vi "main_002.vi"() -> ()   [LabVIEW 2017]
uses:
  ISEGNHQxxu/iseg NHQ VISA Control.ctl
  <vilib>/Analysis/1siggen.llb/Ramp Pattern by Samples.vi
  <vilib>/Utility/file.llb/Read From Spreadsheet File (DBL).vi
  <vilib>/Utility/file.llb/Write Delimited Spreadsheet (string).vi
  <vilib>/Utility/file.llb/Write Delimited Spreadsheet (DBL).vi
  <vilib>/Platform/browser.llb/Open URL in Default Browser (path).vi
  <vilib>/Analysis/NI_AALBase.lvlib
  Newport ESP301/Newport ESP301.lvlib
panel:
  in  "continous acq.":bool
  in  "snap":bool
  in  "dark":bool
  in  "savebin":bool
  in  "savepng":bool
  in  "count?":bool
  in  "dark?":bool=TRUE
  in  "threshold":i32=300
  in  "t_exp":dbl=0.10000637173652649 caption="Exposure time [s]"
  in  "dark_load":bool
  in  "frames":i32=300
  in  "avg[t] acc[f]":bool
  in  "Value in":dbl=2.0 caption="binning"
  in  "stop":bool
  out "Slide":dbl(slide)=0.9966666666666667 scale=0.0..1.0
  in  "open base path":bool
  in  "Path":path=path "Z:/Ediff/data/2018/08/180807"
  in  "Tab Control":T1(tab)=enum."delayscan"
  out "Waveform Chart":dbl(graph)=8402498.700000005
  in  "array size":i32=50
  out "noise-o-meter":dbl=7.252741087138157 format="%.1g"
  out "Actual Voltage":dbl[unit]=-90.03 format="%.2f"
  in  "volt_set":bool
  in  "Nominal Voltage":sgl=90.0 min=0 max=1000 step=1 format="%.2f"
  in  "delayscan_go":bool
  in  "waypoints":string[][](table)=[["-500", "50"], ["500", ""], ["", ""]]
  in  "delayscan_header":string="DelayScan01" caption="header"
  in  "iterations":i32=1
  out "XY Graph":cluster{"Array":dbl[], dbl[]}(graph)={"Array"=[-500.0, -450.0, -400.0, -350.0, -300.0, -250.0, -200.0, -150.0, -100.0, -50.0, 0.0, 50.0, 100.0, 150.0, 200.0, 250.0, 300.0, 350.0, 400.0, 450.0, 500.0], [74.7680418855, 74.77553669695, 0.0, 0.0, 0.0, 0.0, 0.0, 0.0, 0.0, 0.0, 0.0, 0.0, 0.0, 0.0, 0.0, 0.0, 0.0, 0.0, 0.0, 0.0, 0.0]}
  in  "delayscan_stop":bool
  in  "esp_abs_dest":dbl=74.87296924580001 caption="[mm]"
  out "t0 @":dbl=74.84299 format="%.6g"
  in  "esp_set_t0":bool
  in  "esp_abs_time":dbl=200.0 caption="[fs]"
  in  "esp_rel_delta":dbl=0.015 caption="delta [mm]" min=0.0
  in  "esp_abs_go":bool
  in  "esp_rel-":bool
  in  "esp_rel+":bool
  out "delay_pos":dbl=74.77555 caption="[mm]" format="%.6g"
  out "esp_pos_fs":dbl=-449.91125160329966 caption="[fs]" format="%.6g"
  out "Slide 2":dbl(slide)=0.999 scale=0.0..1.0
  in  "meas_stop_volt":bool
  in  "meas_start_volt":bool
  in  "head":string="PowerVoltScan1"
  in  "volt_start":dbl format="%0.2f"
  in  "volt_end":dbl=1.0 format="%0.2f"
  in  "volt_samples":i32=128
  in  "move2com":bool
  in  "meas_start_XY":bool
  in  "showcom":bool
  in  "VISA ISEG":refnum<visa-resource-name>="COM3"
  in  "Channel (A)":enum16{"A", "B"}(ring)=enum."B"
  out "error out":errorcluster
  in  "volt_timeout":u32=6000
  in  "volt_threshold":sgl=2.0 max=4000 format="%.2f"
  in  "esp_axis":i32=1 caption="ESP Axis" min=1 max=3
  in  "esp_visa":refnum<visa-resource-name>="COM2" caption="ESP VISA"
  out "esp301":errorcluster
  in  "Serial Link (RS232)":enum16{"RS232", "USB"}(ring)
  out "captured":dbl[][](graph)
  out "live":dbl[][](graph)
  in  "close":bool
  # "camera"
  # "voltage supply"
  # "Move absolute"
  # "Move relative"
  # "Axis1"
  # "Axis2"
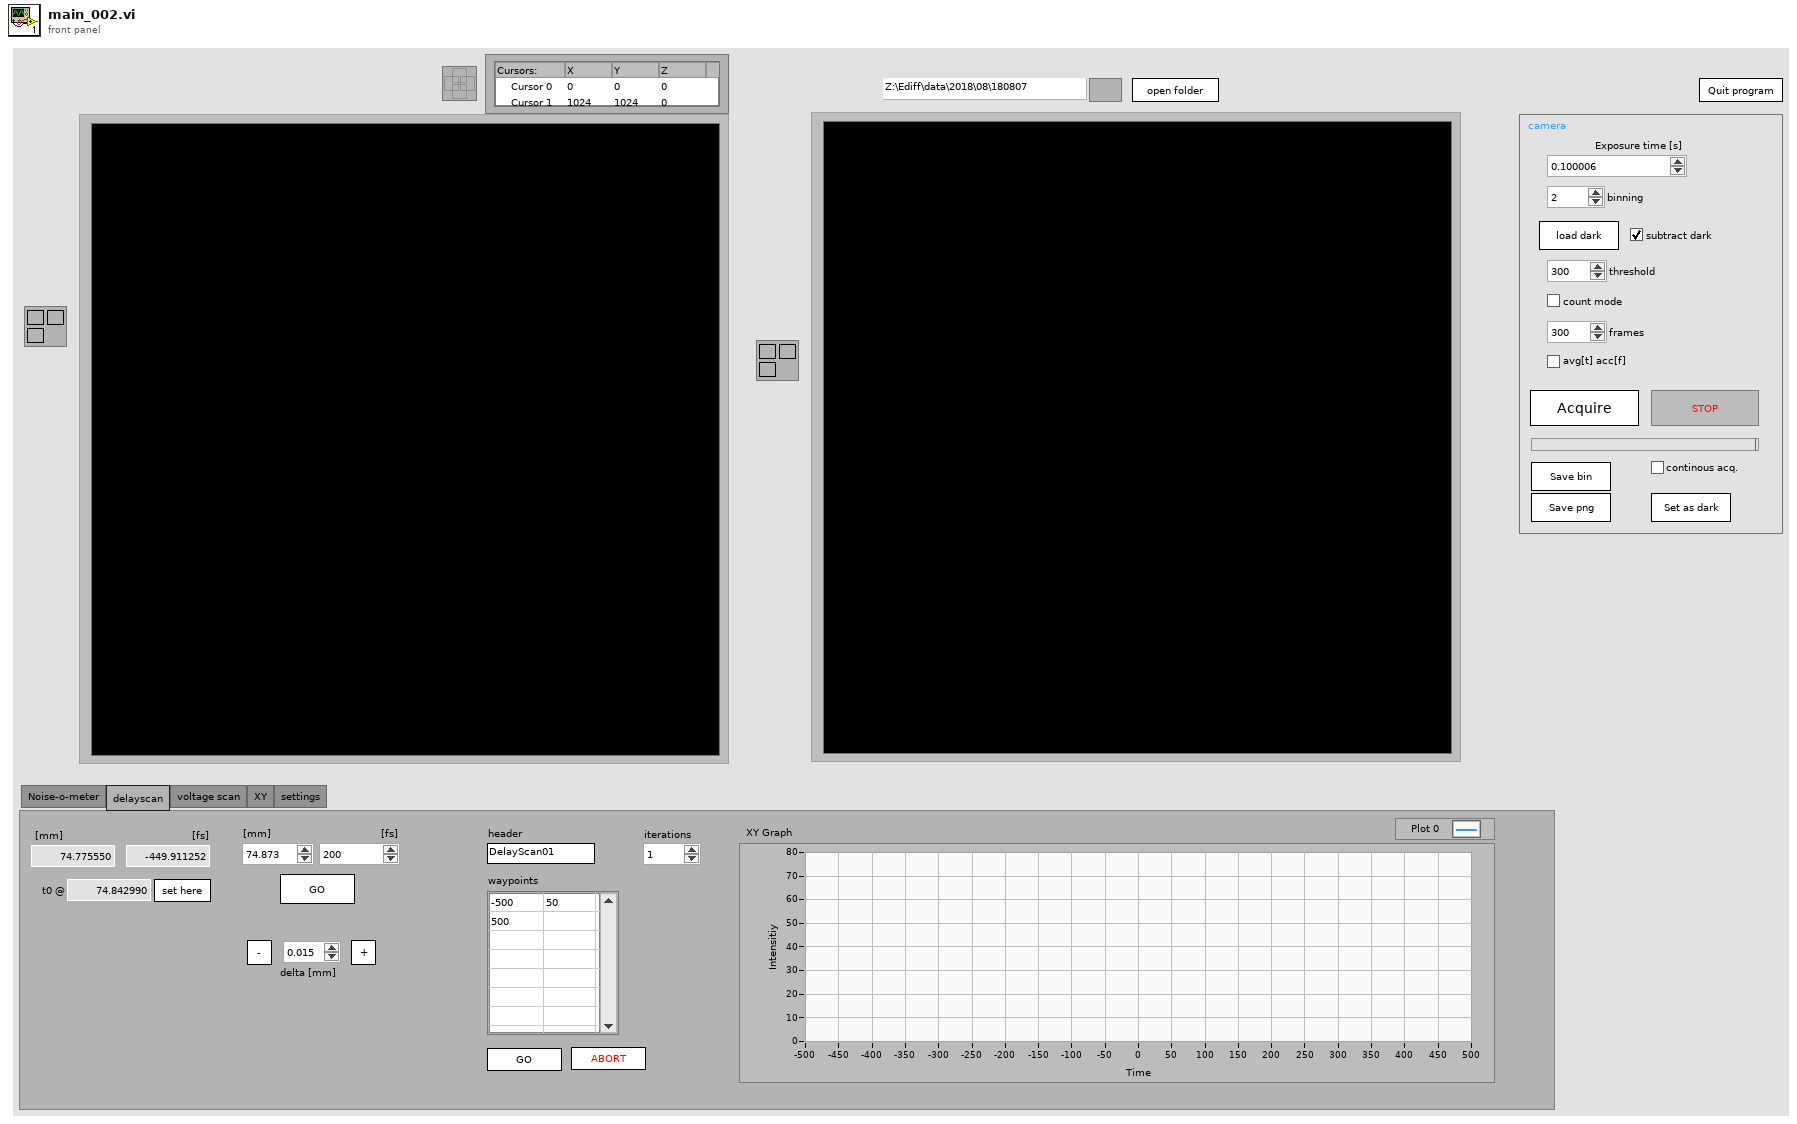
[diagram p1: front panel]
types:
  T1 = enum32{"Noise-o-meter", "delayscan", "voltage scan", "XY", "settings"}
  T2 = typedef "Image Type" = u32
  T3 = typedef "IMAQ Image.ctl" = refnum<image>
  T4 = cluster{"height":u32, "width":u32, "datatype":u32}
  T5 = cluster{"Axis1 moving":bool, "Axis2 moving":bool, "Axis3 moving":bool, "Axis4 moving":bool, "Motor Power of at least one axis":bool, "Reserved":bool, "Reserved":bool, "Reserved":bool, "Axis5 moving 2":bool, "Axis6 moving 2":bool, "Reserved":bool, "Reserved":bool, "Motor Power of at least one axis":bool, "Reserved":bool, "Reserved":bool, "Reserved":bool}
  T6 = typedef "iseg NHQ VISA Control.ctl" = cluster{"VISA Resource Name":refnum<visa-resource-name>, "FP Notation":bool, "Maximum Voltage":u32, "Maximum Current":u32}
  T7 = typedef "LVCursorListTypeDef.ctl" = cluster{"Name":string, "Color":u32, "Style":u8, "Point Style":u8, "Name Visible":bool, "Allow Drag":bool, "Cursor Mode":u32, "Plot":i32, "Index":i32, "Position":cluster{"X":dbl, "Y":dbl}, "X Scale":u32, "Y Scale":u32, "Watch Plots":i32[], "Watch All Plots":bool, "Plot Area":i32, "Label Offset":cluster{"X":dbl, "Y":dbl}}[]
  T8 = cluster{"Name":string, "Color":u32, "Style":u8, "Point Style":u8, "Name Visible":bool, "Allow Drag":bool, "Cursor Mode":u32, "Plot":i32, "Index":i32, "Position":cluster{"X":dbl, "Y":dbl}, "X Scale":u32, "Y Scale":u32, "Watch Plots":i32[], "Watch All Plots":bool, "Plot Area":i32, "Label Offset":cluster{"X":dbl, "Y":dbl}}
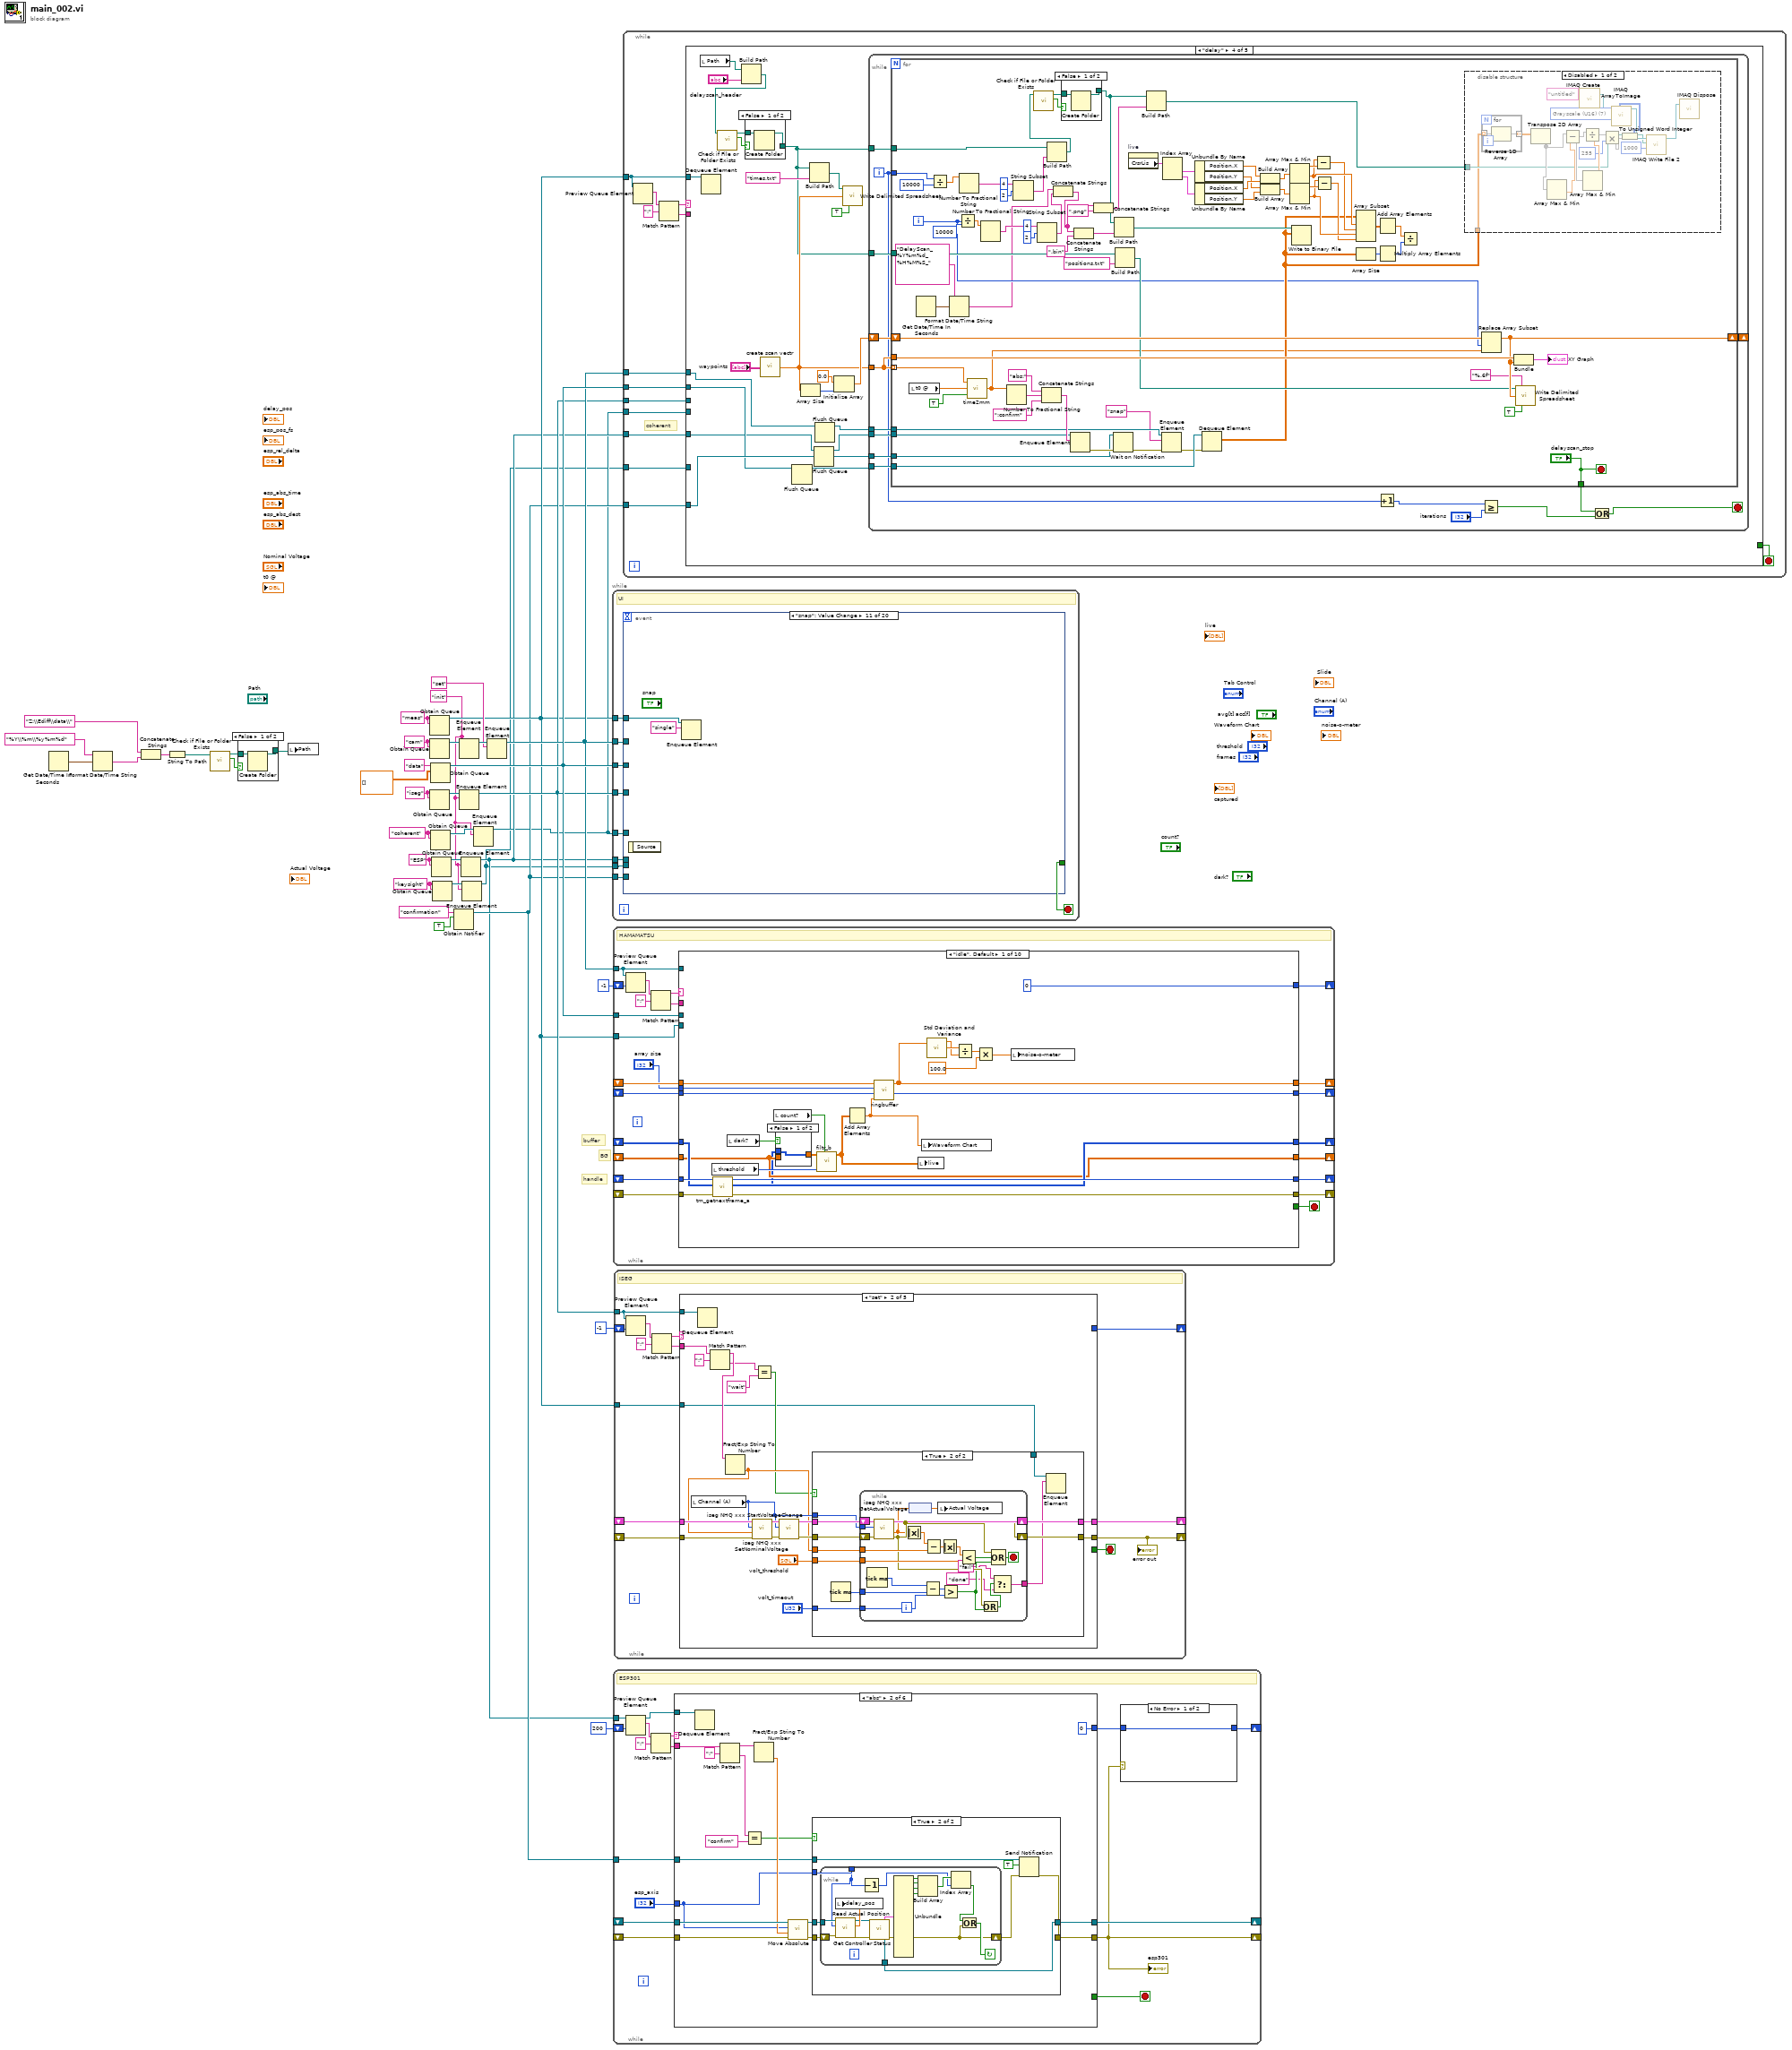
[diagram p0: block diagram]
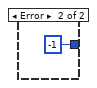
[diagram p3: hidden frame]
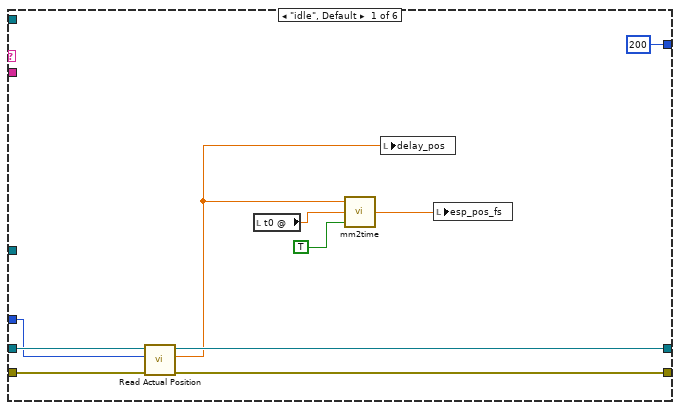
[diagram p4: hidden frame]
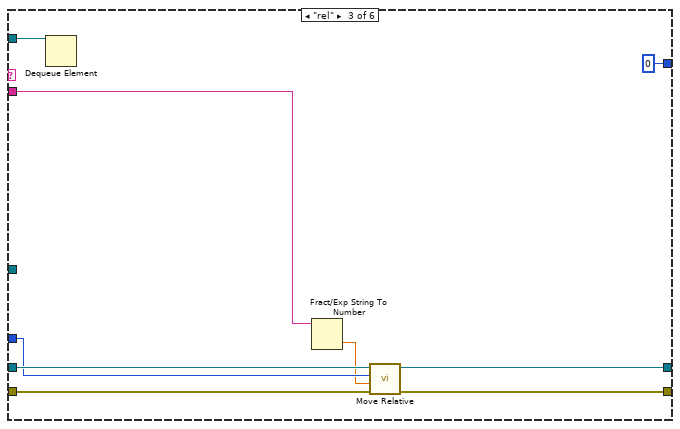
[diagram p6: hidden frame]
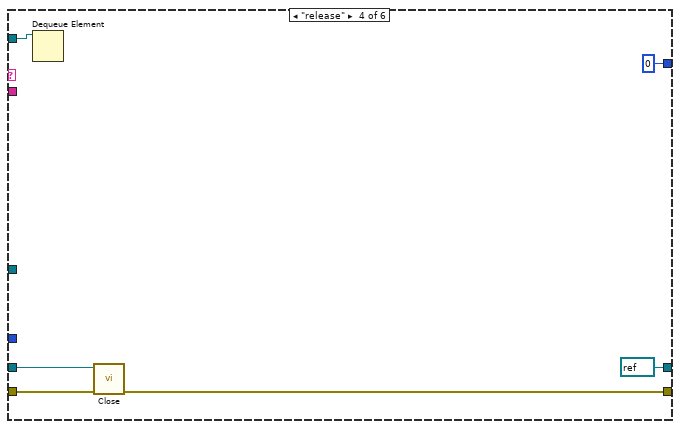
[diagram p7: hidden frame]
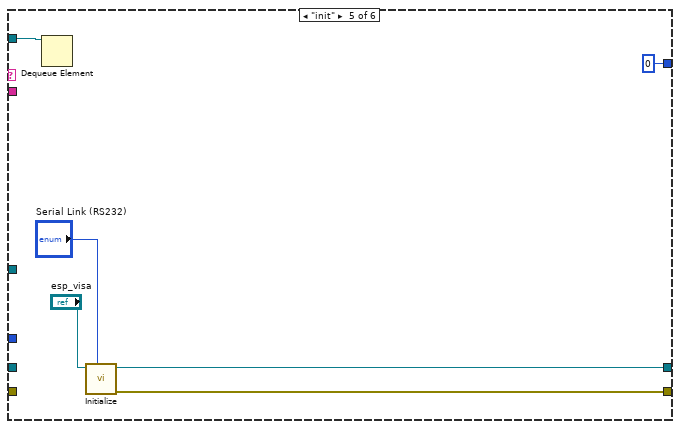
[diagram p8: hidden frame]
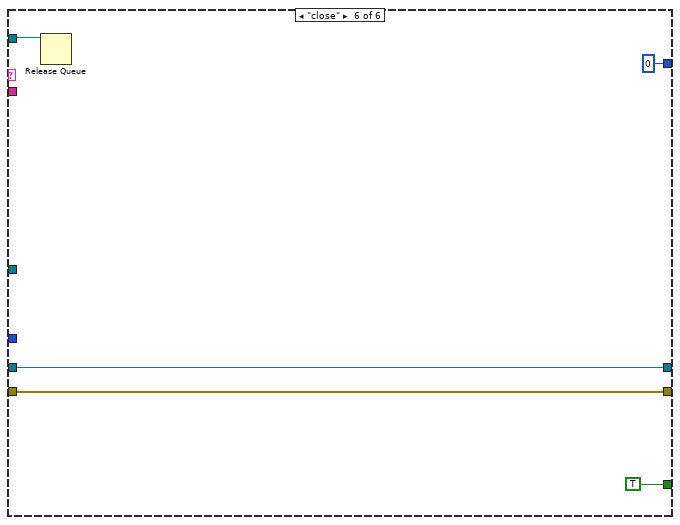
[diagram p9: hidden frame]
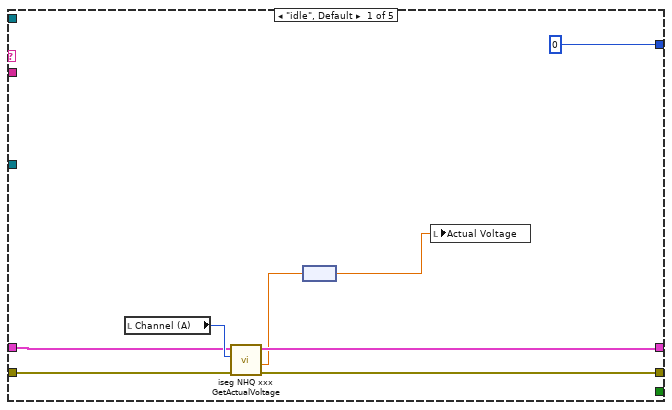
[diagram p10: hidden frame]
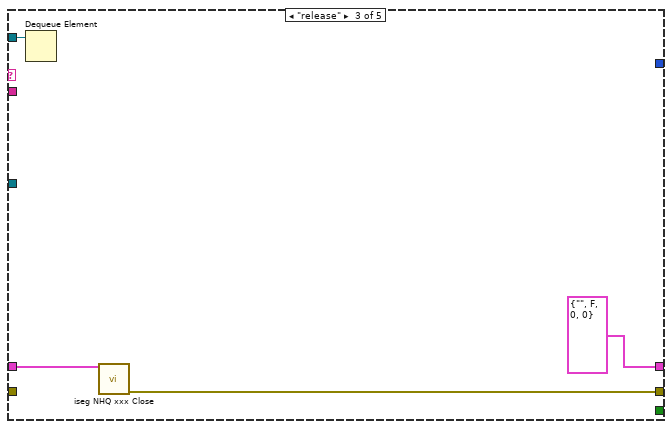
[diagram p12: hidden frame]
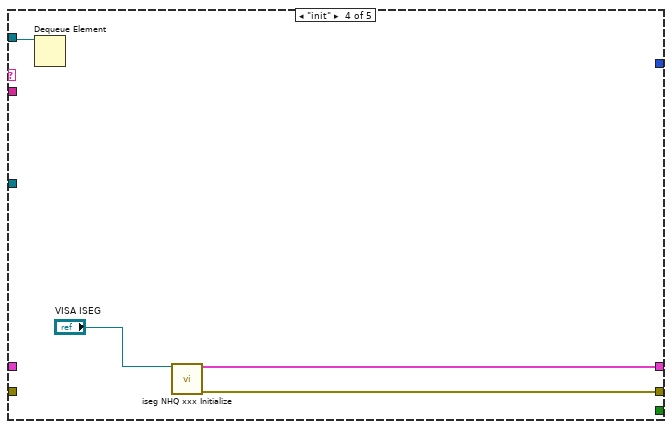
[diagram p13: hidden frame]
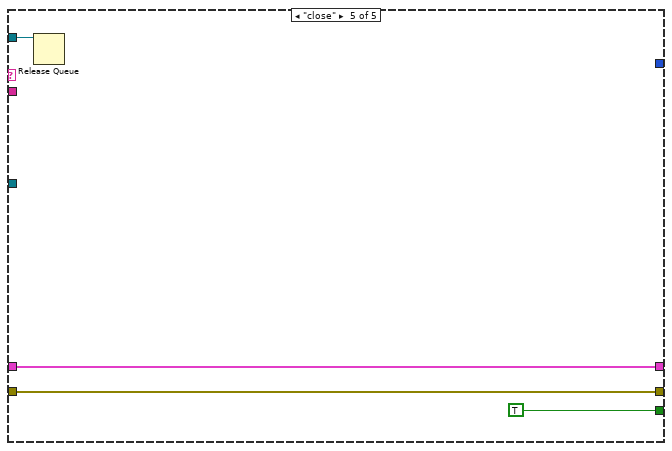
[diagram p14: hidden frame]
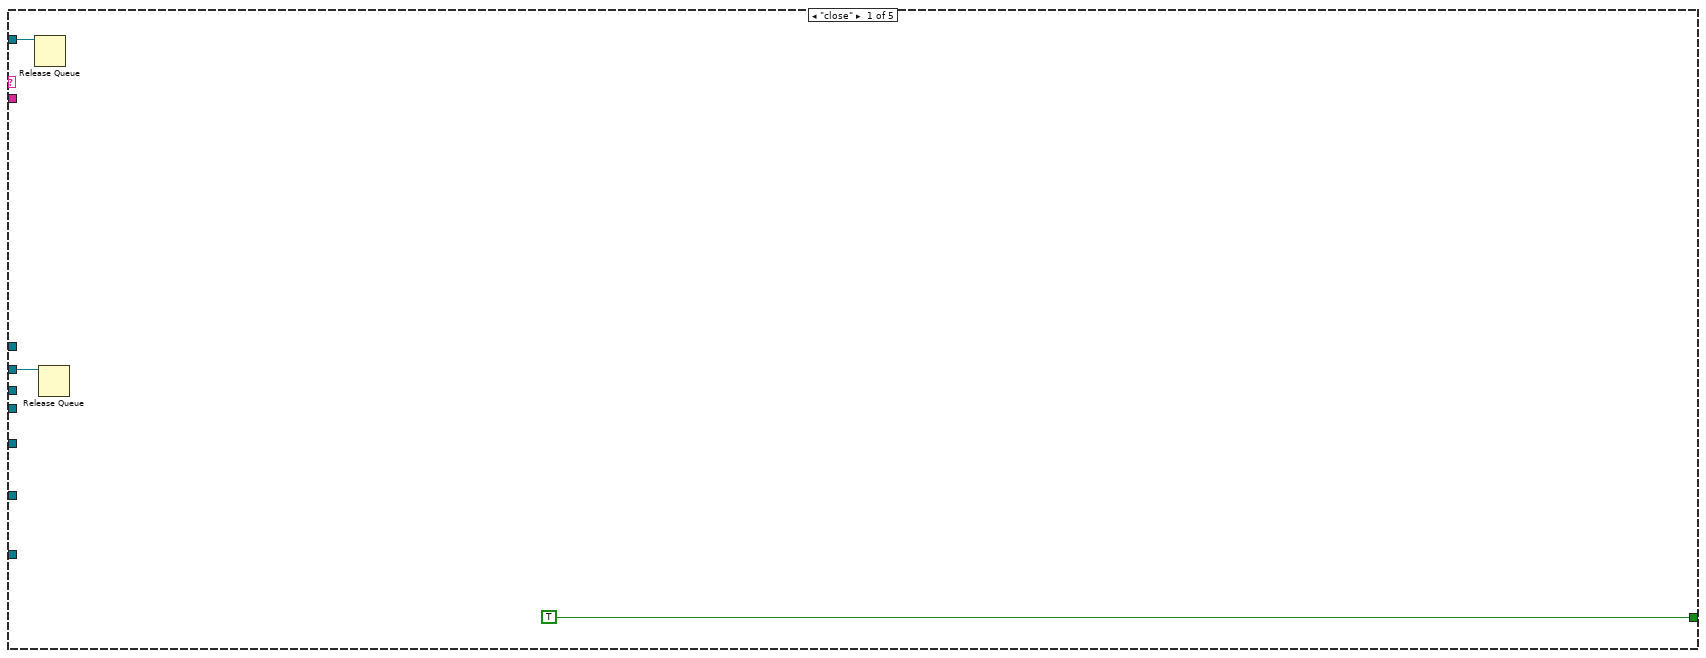
[diagram p15: hidden frame]
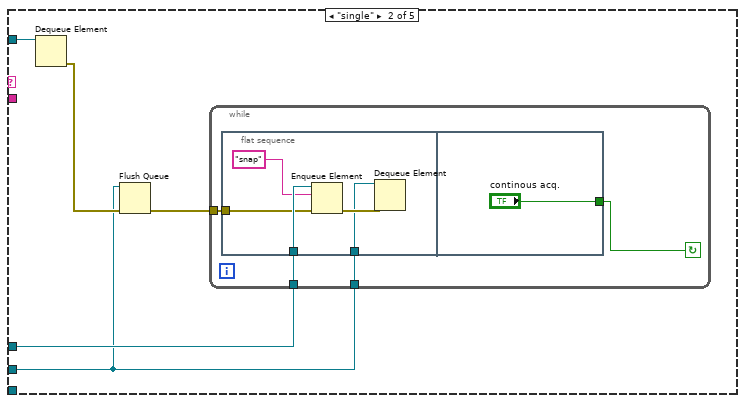
[diagram p16: hidden frame]
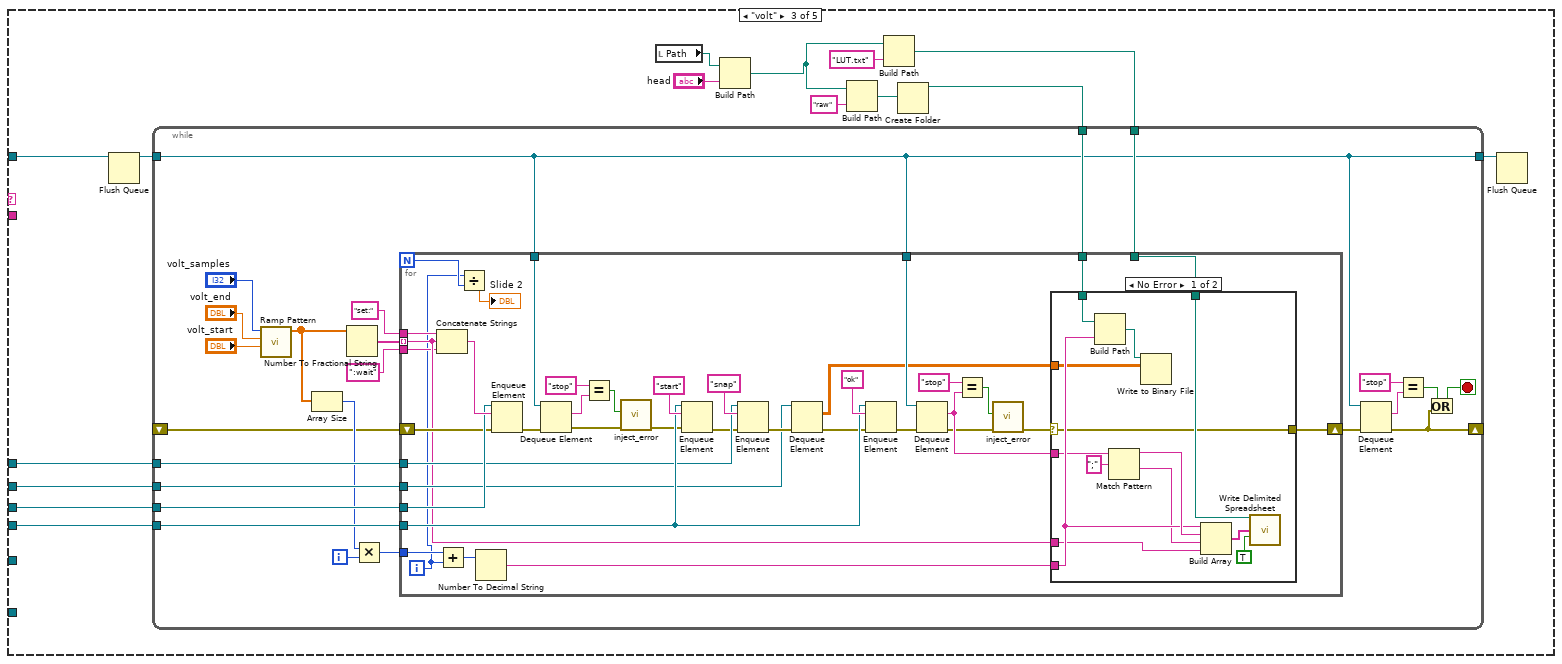
[diagram p17: hidden frame]
diagram:
  w3 = "keysight" ("name (unnamed)")
  w19 = "ESP" ("name (unnamed)")
  w24 = "coherent" ("name (unnamed)")
  w28 = "iseg" ("name (unnamed)")
  w2 = "init" ("element")
  w35 = "meas" ("name (unnamed)")
  w36 = "cam" ("name (unnamed)")
  # "BG"
  # "handle"
  # "buffer"
  n1 = Get Date/Time In Seconds() -> (seconds since 1Jan1904=w16:timestamp)
  n2 = Format Date/Time String(time format string (%c)="%Y\\%m\\%y%m%d", seconds (now)=w16) -> (date/time string=w14:string)  [unwired: 1 in]
  n3 = Concatenate Strings("Z:\\Ediff\\data\\" ("string"), w14) -> (w12:string)
  n4 = String To Path(string=w12) -> (path=w9:path)
  n5 = call <vilib>:"Check if File or Folder Exists.vi"("path"=w9) -> ("file or folder exists?"=w11:bool, "dup path"=w10:path)  [unwired: 8 in, 1 out]
  n6 = case shown="False" w11 {
    tunnel: [w40 w41] -> w8
    tunnel: w10 -> [w39 w41]
    frame False {
      n7 = Create Folder(path (use dialog)=w39) -> (created path=w40:path)  [unwired: 2 in, 2 out]
    }
    frame True {
    }
  }
  n8 = local write "Path"(w8) -> ()
  n9 = Obtain Queue(name (unnamed)=w35, element data type=w35) -> (queue out=w23:refnum<queue>)  [unwired: 3 in, 2 out]
  n10 = Obtain Queue(name (unnamed)=w36, element data type=w36) -> (queue out=w38:refnum<queue>)  [unwired: 3 in, 2 out]
  n11 = Obtain Queue(name (unnamed)=w28, element data type=w28) -> (queue out=w27:refnum<queue>)  [unwired: 3 in, 2 out]
  n12 = Obtain Queue(name (unnamed)="data", element data type=dbl[][] []) -> (queue out=w31:refnum<queue>)  [unwired: 3 in, 2 out]
  n13 = Obtain Queue(name (unnamed)=w24, element data type=w24) -> (queue out=w7:refnum<queue>)  [unwired: 3 in, 2 out]
  n14 = Obtain Queue(name (unnamed)=w19, element data type=w19) -> (queue out=w18:refnum<queue>)  [unwired: 3 in, 2 out]
  n15 = Obtain Queue(name (unnamed)=w3, element data type=w3) -> (queue out=w4:refnum<queue>)  [unwired: 3 in, 2 out]
  n16 = Obtain Notifier(name (unnamed)="confirmation", notification data type=TRUE) -> (notifier out=w20:refnum<notifier>)  [unwired: 2 in, 2 out]
  n17 = Enqueue Element(queue=w38, element=w2) -> (queue out=w34:refnum<queue>)  [unwired: 2 in, 2 out]
  n18 = Enqueue Element(queue=w27, element=w2) -> (queue out=w25:refnum<queue>)  [unwired: 2 in, 2 out]
  n19 = Enqueue Element(queue=w18, element=w2) -> (queue out=w17:refnum<queue>)  [unwired: 2 in, 2 out]
  n20 = Enqueue Element(queue=w4, element=w2) -> (queue out=w1:refnum<queue>)  [unwired: 2 in, 2 out]
  n21 = Enqueue Element(queue=w7, element=w2) -> (queue out=w6:refnum<queue>)  [unwired: 2 in, 2 out]
  n22 = Enqueue Element(queue=w34, element="set") -> (queue out=w30:refnum<queue>)  [unwired: 2 in, 2 out]
  n23 = while {
    tunnel: w30 -> [w50]
    tunnel: w23 -> [w49]
    tunnel: w31 -> [w48]
    tunnel: w25 -> [w46]
    tunnel: w6 -> [w45]
    tunnel: w20 -> [w44]
    tunnel: w17 -> [w43]
    tunnel: w1 -> [w42]
    stop <- w47 stop-if-true
    # "UI"
    n24 = event shown="[10] \"snap\": Value Change" {
      selector: _ -> [_ _ _ _ _ _ _ _ _ _ _ _ _ _ _ _ _ _ _ _]
      dyn-events: _ -> [_ _ _ _ _ _ _ _ _ _ _ _ _ _ _ _ _ _ _ _]
      timeout: _ -> [_ _ _ _ _ _ _ _ _ _ _ _ _ _ _ _ _ _ _ _]
      tunnel: w50 -> [_ w65 _ _ _ _ _ _ w93 w95 _ _ _ _ _ _ w146 _ _ _]
      tunnel: w49 -> [_ w66 _ _ _ _ w87 _ _ _ w96 w99 w100 _ _ w140 _ w153 w155 _]
      tunnel: w48 -> [_ _ _ _ _ _ _ _ _ _ _ _ _ _ _ _ _ _ _ _]
      tunnel: [_ TRUE _ _ _ _ _ _ _ _ _ _ _ _ _ _ _ _ _ _] -> w47
      tunnel: w46 -> [_ w62 _ _ _ _ _ _ _ _ _ _ _ _ _ _ _ _ _ w160]
      tunnel: w45 -> [_ w59 _ _ _ _ _ _ _ _ _ _ _ _ _ _ _ _ _ _]
      tunnel: w44 -> [_ w56 _ _ _ _ _ _ _ _ _ _ _ _ _ _ _ _ _ _]
      tunnel: w43 -> [_ w58 w72 w77 _ _ _ _ _ _ _ _ _ _ _ _ _ _ _ _]
      tunnel: w42 -> [_ w51 _ _ _ _ _ _ _ _ _ _ _ _ _ _ _ _ _ _]
      event Timeout {
        n25 = event-data() -> ()  [unwired: 1 in, 1 out]
      }
      event "close": Value Change {
        w54 = "close" ("element")
        w55 = "release" ("element")
        n26 = event-data() -> ()  [unwired: 1 in, 1 out]
        n27 = Enqueue Element(queue=w59, element=w55) -> (queue out=w60:refnum<queue>)  [unwired: 2 in, 2 out]
        n28 = Enqueue Element(queue=w58, element=w55) -> (queue out=w57:refnum<queue>)  [unwired: 2 in, 2 out]
        n29 = Enqueue Element(queue=w62, element=w55) -> (queue out=w61:refnum<queue>)  [unwired: 2 in, 2 out]
        n30 = Enqueue Element(queue=w65, element=w55) -> (queue out=w64:refnum<queue>)  [unwired: 2 in, 2 out]
        n31 = Enqueue Element(queue=w66, element=w54) -> ()  [unwired: 2 in, 3 out]
        n32 = Enqueue Element(queue=w64, element=w54) -> ()  [unwired: 2 in, 3 out]
        n33 = Enqueue Element(queue=w61, element=w54) -> ()  [unwired: 2 in, 3 out]
        n34 = Enqueue Element(queue=w60, element=w54) -> ()  [unwired: 2 in, 3 out]
        n35 = Enqueue Element(queue=w57, element=w54) -> ()  [unwired: 2 in, 3 out]
        n36 = Release Notifier(notifier=w56) -> ()  [unwired: 2 in, 3 out]
        n37 = Flush Queue(queue=w51) -> (queue out=w52:refnum<queue>)  [unwired: 1 in, 2 out]
        n38 = Enqueue Element(queue=w52, element=w55) -> (queue out=w53:refnum<queue>)  [unwired: 2 in, 2 out]
        n39 = Enqueue Element(queue=w53, element=w54) -> ()  [unwired: 2 in, 3 out]
      }
      event "esp_abs_go": Value Change {
        n40 = event-data() -> ()  [unwired: 1 in, 1 out]
        n41 = local read "esp_abs_dest"() -> (w68:dbl)
        n42 = Number To Fractional String(number=w68) -> (F-format string=w69:string)  [unwired: 3 in]
        n43 = Concatenate Strings("abs:" ("string"), w69, ":confirm" ("string")) -> (w71:string)
        n44 = Enqueue Element(queue=w72, element=w71) -> ()  [unwired: 2 in, 3 out]
      }
      event "esp_rel+", "esp_rel-": Value Change {
        n45 = event-data() -> ()  [unwired: 1 in, 1 out]
        n46 = local read "esp_rel_delta"() -> (w75:dbl)
        n47 = Negate(x=w75) -> (-x=w76:dbl)
        n48 = Select(t=w76, s="esp_rel-", f=w75) -> (s? t:f=w74:dbl)
        n49 = Number To Fractional String(number=w74) -> (F-format string=w79:string)  [unwired: 3 in]
        n50 = Concatenate Strings("rel:" ("string"), w79) -> (w78:string)
        n51 = Enqueue Element(queue=w77, element=w78) -> ()  [unwired: 2 in, 3 out]
      }
      event "esp_set_t0": Value Change {
        n52 = event-data() -> ()  [unwired: 1 in, 1 out]
        n53 = local read "delay_pos"() -> (w81:dbl)
        n54 = local write "t0 @"(w81) -> ()
      }
      event "esp_abs_time": Value Change {
        n55 = event-data() -> ()  [unwired: 1 in, 1 out]
        n56 = local read "esp_abs_time"() -> (w82:dbl)
        n57 = local read "t0 @"() -> (w83:dbl)
        n58 = call "time2mm.vi"("fs[1]/ps[0]"=TRUE, "Offset (mm)"=w83, "time"=w82) -> ("position (mm)"=w84:dbl)
        n59 = local write "esp_abs_dest"(w84) -> ()
      }
      event "delayscan_go": Value Change {
        n60 = event-data() -> ()  [unwired: 1 in, 1 out]
        n61 = Enqueue Element(queue=w87, element="delay") -> ()  [unwired: 2 in, 3 out]
      }
      event "esp_abs_dest": Value Change {
        n62 = event-data() -> ()  [unwired: 1 in, 1 out]
        n63 = local read "esp_abs_dest"() -> (w91:dbl)
        n64 = local read "t0 @"() -> (w90:dbl)
        n65 = call "mm2time.vi"("fs?"=TRUE, "Offset (mm)"=w90, "distance (mm)"=w91) -> ("time in fs/ps seconds"=w88:dbl)
        n66 = local write "esp_abs_time"(w88) -> ()
      }
      event "dark": Value Change {
        n67 = event-data() -> ()  [unwired: 1 in, 1 out]
        n68 = Enqueue Element(queue=w93, element="dark") -> ()  [unwired: 2 in, 3 out]
      }
      event "t_exp": Value Change {
        n69 = event-data() -> ()  [unwired: 1 in, 1 out]
        n70 = Enqueue Element(queue=w95, element="set") -> ()  [unwired: 2 in, 3 out]
      }
      event "snap": Value Change {
        n71 = event-data() -> ()  [unwired: 1 in, 1 out]
        n72 = Enqueue Element(queue=w96, element="single") -> ()  [unwired: 2 in, 3 out]
      }
      event "meas_start_volt": Value Change {
        n73 = event-data() -> ()  [unwired: 1 in, 1 out]
        n74 = Enqueue Element(queue=w99, element="volt") -> ()  [unwired: 2 in, 3 out]
      }
      event "meas_stop_volt": Value Change {
        n75 = event-data() -> ()  [unwired: 1 in, 1 out]
        n76 = Enqueue Element(queue=w100, element="stop") -> ()  [unwired: 2 in, 3 out]
      }
      event "open base path": Value Change {
        n77 = event-data() -> ()  [unwired: 1 in, 1 out]
        n78 = local read "Path"() -> (w102:path)
        n79 = call-poly <vilib>:"Open URL in Default Browser.vi"("path"=w102) -> ()  [unwired: 5 in, 2 out]
      }
      event "savebin", "savepng": Value Change {
        n80 = event-data() -> ()  [unwired: 1 in, 1 out]
        n81 = Get Date/Time In Seconds() -> (seconds since 1Jan1904=w108:timestamp)
        n82 = local read "Path"() -> (w104:path)
        n83 = Format Date/Time String(time format string (%c)="MCPIMG_%Y%m%d_%H%M%S", seconds (now)=w108) -> (date/time string=w103:string)  [unwired: 1 in]
        n84 = local read "captured"() -> (w105:dbl[][])
        n85 = case shown="False" "savebin" {
          tunnel: w105 -> [w123 w139]
          tunnel: w104 -> [w120 w133]
          tunnel: w103 -> [w118 w134]
          frame False {
            w128 = T2 7 items=["Grayscale (U8)", "Grayscale (I16)", "Grayscale (SGL)", "Complex (CSG)", "RGB (U32)", "HSL (U32)", "RGB (U64)", "Grayscale (U16)"] ("Image Type")
            n86 = for {
              tunnel: w123 -> [w131] mode=indexing
              tunnel: [w130] -> w122 mode=indexing
              n87 = Reverse 1D Array(array=w131) -> (reversed array=w130:dbl[])
            }
            n88 = Concatenate Strings(w118, ".png" ("string")) -> (w119:string)
            n89 = Transpose 2D Array(2D array=w122) -> (transposed array=w111:dbl[][])
            n90 = Array Max & Min(array=w111) -> (min value=w110:dbl)  [unwired: 3 out]
            n91 = Build Path(base path=w120, name or relative path=w119) -> (appended path=w121:path)
            n92 = Subtract(x=w111, y=w110) -> (x-y=w109:dbl[][])
            n93 = call "IMAQ Create"("Image Name"="untitled", "Image Type"=w128) -> ("New Image"=w129:T3)  [unwired: 3 in, 1 out]
            n94 = Array Max & Min(array=w109) -> (max value=w116:dbl)  [unwired: 3 out]
            n95 = Divide(x=w109, y=w116) -> (x/y=w115:dbl[][])
            n96 = Multiply(x=w115, y=255) -> (x*y=w113:dbl[][])
            n97 = To Unsigned Word Integer(number=w113) -> (unsigned 16bit integer=w112:u16[][])
            n98 = call "IMAQ ArrayToImage"("Image Pixels (U16)"=w112, "Image"=w129) -> ("Image Out"=w127:T3)  [unwired: 8 in, 1 out]
            n99 = call-poly "IMAQ Write File 2"("Image Quality"=u32 1000, "File Path"=w121, "Image"=w127) -> ("Image Out (duplicate)"=w125:T3)  [unwired: 7 in, 1 out]
            n100 = call "IMAQ Dispose"("Image"=w125) -> ()  [unwired: 5 in, 1 out]
          }
          frame True {
            n101 = Concatenate Strings(w134, ".bin" ("string")) -> (w136:string)
            n102 = Build Path(base path=w133, name or relative path=w136) -> (appended path=w132:path)
            n103 = Write to Binary File(file (use dialog)=w132, data=w139) -> (refnum out=w138:refnum<file>, error out=w137:errorcluster)  [unwired: 4 in, 1 out]
            n104 = Close File(refnum=w138, error in=w137) -> ()  [unwired: 2 out]
          }
        }
      }
      event "meas_start_XY": Value Change {
        n105 = event-data() -> ()  [unwired: 1 in, 1 out]
        n106 = Enqueue Element(queue=w140, element="XY") -> ()  [unwired: 2 in, 3 out]
      }
      event "dark_load": Value Change {
        n107 = event-data() -> ()  [unwired: 1 in, 1 out]
        n108 = local read "Path"() -> (w145:path)
        n109 = call "File Dialog"("start path"=w145) -> ("selected path"=w143:path, "cancelled"=w142:bool)  [unwired: 11 in, 2 out]
        n110 = case shown="False" w142 {
          tunnel: w146 -> [w151 _]
          tunnel: "dark_load:" ("element") -> [w149 _]
          tunnel: w143 -> [w147 _]
          frame False {
            n111 = Path To String(path=w147) -> (string=w148:string)
            n112 = Concatenate Strings(w149, w148) -> (w150:string)
            n113 = Enqueue Element(queue=w151, element=w150) -> ()  [unwired: 2 in, 3 out]
          }
          frame True {
          }
        }
      }
      event "move2com": Value Change {
        n114 = event-data() -> ()  [unwired: 1 in, 1 out]
        n115 = Enqueue Element(queue=w153, element="mov2cursor") -> ()  [unwired: 2 in, 3 out]
      }
      event "showcom": Value Change {
        n116 = event-data() -> ()  [unwired: 1 in, 1 out]
        n117 = Enqueue Element(queue=w155, element="showcom") -> ()  [unwired: 2 in, 3 out]
      }
      event "volt_set": Value Change {
        n118 = event-data() -> ()  [unwired: 1 in, 6 out]
        n119 = local read "Nominal Voltage"() -> (w156:sgl)
        n120 = Number To Fractional String(number=w156) -> (F-format string=w157:string)  [unwired: 3 in]
        n121 = Concatenate Strings("set:" ("element"), w157) -> (w159:string)
        n122 = Enqueue Element(queue=w160, element=w159) -> ()  [unwired: 2 in, 3 out]
      }
    }
  }
  n123 = while {
    tunnel: w30 -> [w179]
    shift-right: [w177] -> _
    shift-left: _ -> [w176]
    shift-right: [w175] -> _
    shift-left: _ -> [w174]
    shift-right: [w173] -> _
    shift-left: _ -> [w172]
    shift-right: [w171] -> _
    shift-left: _ -> [w170]
    shift-right: [w168] -> _
    shift-left: -1 -> [w169]
    tunnel: w31 -> [w167]
    tunnel: w23 -> [w166]
    shift-right: [w165] -> _
    shift-left: _ -> [w164]
    shift-right: [w162] -> _
    shift-left: _ -> [w163]
    stop <- w178 stop-if-true
    # "HAMAMATSU"
    n124 = Preview Queue Element(queue=w179, timeout in ms (-1)=w169) -> (element=w183:string)  [unwired: 1 in, 3 out]
    n125 = Match Pattern(string=w183, regular expression=":") -> (before substring=w181:string, after substring=w180:string)  [unwired: 1 in, 2 out]
    n126 = case shown="\"idle\", Default" w181 {
      tunnel: w180 -> [_ _ w283 _ _ w373 _ _ _ _]
      tunnel: w179 -> [_ w222 w284 w318 w367 w377 w389 w392 w418 w440]
      tunnel: [_ _ _ _ _ _ _ _ _ TRUE] -> w178
      tunnel: [w202 w224 w287 w323 w365 w374 w381 w397 w406 w435] -> w177
      tunnel: w176 -> [w204 w227 w289 w325 w365 w374 w385 _ w432 w435]
      tunnel: [w203 w219 w288 w322 w364 w375 u32 0 ("Handle out") w395 w407 w436] -> w175
      tunnel: w174 -> [w205 w225 w290 w326 w364 w375 w386 _ w430 w436]
      tunnel: [w201 w226 w282 w321 w366 w376 w387 w393 w419 w437] -> w173
      tunnel: w172 -> [w201 w226 w282 w321 w366 w376 w387 w393 _ w437]
      tunnel: [w200 w223 w291 w324 w363 w370 w388 w394 w410 w438] -> w171
      tunnel: w170 -> [w200 w223 w291 w324 _ _ w388 w394 w410 w438]
      tunnel: [0 _ _ _ _ _ _ _ _ _] -> w168
      tunnel: w167 -> [_ w218 w292 _ _ _ _ _ _ _]
      tunnel: w166 -> [_ _ _ w319 _ _ _ _ _ _]
      tunnel: [w186 w213 w286 w310 w362 w369 w379 w391 w412 w434] -> w165
      tunnel: w164 -> [w195 w216 w286 w313 w362 w369 w379 w391 w412 w434]
      tunnel: w163 -> [w190 w215 w285 w311 w361 w368 w378 w390 w411 w433]
      tunnel: [w189 w212 w285 w309 w361 w368 w378 w390 w411 w433] -> w162
      tunnel: "array size" -> [w188 w214 _ w312 _ _ _ _ _ _]
      frame "idle", Default {
        n127 = local read "threshold"() -> (w206:i32)
        n128 = call "tm_getnextframe_a.vi"("error in (no error)"=w204, "Buffer"=w201, "Handle in"=w205) -> ("error out"=w202:errorcluster, "Data"=w196:u16[][], "Handle out"=w203:u32)  [unwired: 6 in]
        n129 = local read "dark?"() -> (w207:bool)
        n130 = local read "count?"() -> (w197:bool)
        n131 = case shown="False" w207 {
          tunnel: [w208 w211] -> w198
          tunnel: w196 -> [w208 w210]
          tunnel: w200 -> [_ w209]
          frame False {
          }
          frame True {
            n132 = Subtract(x=w210, y=w209) -> (x-y=w211:dbl[][])
          }
        }
        n133 = call "filtr_b.vi"("count?"=w197, "threshold"=w206, "input array"=w198) -> ("output array"=w184:dbl[][])  [unwired: 8 in]
        n134 = Add Array Elements(numeric array=w184) -> (sum=w185:dbl)
        n135 = call "ringbuffer.vi"("new val"=w185, "index in"=w190, "array size"=w188, "array in"=w195) -> ("index out"=w189:i32, "array out"=w186:dbl[])  [unwired: 6 in]
        n136 = local write "live"(w184) -> ()
        n137 = local write "Waveform Chart"(w185) -> ()
        n138 = call <vilib>:"Std Deviation and Variance.vi"("X"=w186) -> ("mean"=w191:dbl, "standard deviation"=w194:dbl)  [unwired: 1 in, 1 out]
        n139 = Divide(x=w194, y=w191) -> (x/y=w193:dbl)
        n140 = Multiply(x=w193, y=100.0) -> (x*y=w187:dbl)
        n141 = local write "noise-o-meter"(w187) -> ()
      }
      frame "snap" {
        n142 = Dequeue Element(queue=w222) -> ()  [unwired: 2 in, 4 out]
        n143 = local read "avg[t] acc[f]"() -> (w221:bool)
        n144 = local read "threshold"() -> (w229:i32)
        n145 = local read "frames"() -> (w228:i32)
        n146 = local read "count?"() -> (w220:bool)
        n147 = local read "dark?"() -> (w230:bool)
        n148 = for {
          N: w228 -> [w248]
          tunnel: w230 -> [w262]
          tunnel: w226 -> [w260]
          tunnel: w225 -> [w261]
          tunnel: w229 -> [w254]
          tunnel: [w258] -> w219
          shift-right: [w257] -> w224
          shift-left: w227 -> [w259]
          tunnel: w223 -> [w253]
          shift-right: [w231] -> w217
          shift-left: w226 -> [w251]
          tunnel: w221 -> [w252]
          tunnel: w220 -> [w250]
          shift-right: [w241] -> w213
          shift-left: w216 -> [w242]
          tunnel: w214 -> [w239]
          shift-right: [w238] -> w212
          shift-left: w215 -> [w240]
          shift-right: [w234] -> _
          shift-left: _ -> [w235]
          i -> [w249]
          stop <- "stop" stop-if-true
          n149 = call "tm_getnextframe_a.vi"("error in (no error)"=w259, "Buffer"=w260, "Handle in"=w261) -> ("error out"=w257:errorcluster, "Data"=w256:u16[][], "Handle out"=w258:u32)  [unwired: 6 in]
          n150 = Divide(x=w249, y=w248) -> (x/y=w247:dbl)
          n151 = case shown="True" w262 {
            tunnel: [w273 w276] -> w255
            tunnel: w256 -> [w273 w275]
            tunnel: w253 -> [_ w274]
            frame False {
            }
            frame True {
              n152 = Subtract(x=w275, y=w274) -> (x-y=w276:dbl[][])
            }
          }
          n153 = local write "Slide"(w247) -> ()
          n154 = Tick Count (ms)() -> (millisecond timer value=w234:u32)
          n155 = call "filtr_b.vi"("count?"=w250, "threshold"=w254, "input array"=w255) -> ("output array"=w233:dbl[][])  [unwired: 8 in]
          n156 = Subtract(x=w234, y=w235) -> ()  [unwired: 1 out]
          n157 = Add Array Elements(numeric array=w233) -> (sum=w232:dbl)
          n158 = call "ringbuffer.vi"("new val"=w232, "index in"=w240, "array size"=w239, "array in"=w242) -> ("index out"=w238:i32, "array out"=w241:dbl[])  [unwired: 6 in]
          n159 = call <vilib>:"Std Deviation and Variance.vi"("X"=w241) -> ("mean"=w243:dbl, "standard deviation"=w245:dbl)  [unwired: 1 in, 1 out]
          n160 = local write "live"(w233) -> ()
          n161 = local write "Waveform Chart"(w232) -> ()
          n162 = Divide(x=w245, y=w243) -> (x/y=w237:dbl)
          n163 = case shown="True" w252 {
            tunnel: w251 -> [w265 w272]
            tunnel: w233 -> [w264 w270]
            tunnel: [w263 w266] -> w231
            tunnel: w249 -> [_ w267]
            frame False {
              n164 = Add(x=w265, y=w264) -> (x+y=w263:dbl[][])
            }
            frame True {
              n165 = Multiply(x=w272, y=w267) -> (x*y=w271:dbl[][])
              n166 = Increment(x=w267) -> (x+1=w268:i32)
              n167 = Add(x=w271, y=w270) -> (x+y=w269:dbl[][])
              n168 = Divide(x=w269, y=w268) -> (x/y=w266:dbl[][])
            }
          }
          n169 = Multiply(x=w237, y=100.0) -> (x*y=w236:dbl)
          n170 = local write "noise-o-meter"(w236) -> ()
          n171 = local write "captured"(w231) -> ()
        }
        n172 = local write "captured"(w217) -> ()
        n173 = Enqueue Element(queue=w218, element=w217) -> ()  [unwired: 2 in, 3 out]
      }
      frame "single" {
        n174 = Dequeue Element(queue=w284) -> ()  [unwired: 2 in, 4 out]
        n175 = Decimal String To Number(string=w283) -> (number=w278:i32)  [unwired: 2 in, 1 out]
        n176 = To Unsigned Quad Integer(1:w282) -> (0:w281:u64[][])
        n177 = for {
          N: w278 -> [_]
          tunnel: w282 -> [w304]
          tunnel: w290 -> [w303]
          tunnel: w289 -> [w302]
          tunnel: [w301] -> w288
          tunnel: [w300] -> w287
          shift-right: [w297] -> w280
          shift-left: w281 -> [w299]
          n178 = call "tm_getnextframe_a.vi"("error in (no error)"=w302, "Buffer"=w304, "Handle in"=w303) -> ("error out"=w300:errorcluster, "Data"=w298:u16[][], "Handle out"=w301:u32)  [unwired: 6 in]
          n179 = Add(x=w298, y=w299) -> (x+y=w297:u64[][])
        }
        n180 = local read "dark?"() -> (w293:bool)
        n181 = Divide(x=w280, y=w278) -> (x/y=w279:dbl[][])
        n182 = case shown="True" w293 {
          tunnel: [w305 w308] -> w296
          tunnel: w279 -> [w305 w307]
          tunnel: w291 -> [_ w306]
          frame False {
          }
          frame True {
            n183 = Subtract(x=w307, y=w306) -> (x-y=w308:dbl[][])
          }
        }
        n184 = local read "threshold"() -> (w294:i32)
        n185 = local read "count?"() -> (w295:bool)
        n186 = call "filtr_b.vi"("count?"=w295, "threshold"=w294, "input array"=w296) -> ("output array"=w277:dbl[][])  [unwired: 8 in]
        n187 = Enqueue Element(queue=w292, element=w277) -> ()  [unwired: 2 in, 3 out]
        n188 = local write "captured"(w277) -> ()
      }
      frame "snap_I" {
        n189 = Dequeue Element(queue=w318) -> ()  [unwired: 2 in, 4 out]
        n190 = local read "threshold"() -> (w329:i32)
        n191 = local read "frames"() -> (w328:i32)
        n192 = local read "count?"() -> (w327:bool)
        n193 = local read "dark?"() -> (w330:bool)
        n194 = for {
          N: w328 -> [w344]
          tunnel: w330 -> [w356]
          tunnel: w321 -> [w354]
          tunnel: w326 -> [w355]
          tunnel: w329 -> [w348]
          tunnel: [w352] -> w322
          shift-right: [w351] -> w323
          shift-left: w325 -> [w353]
          tunnel: w324 -> [w347]
          tunnel: w327 -> [w346]
          tunnel: [w342] -> w320 mode=indexing
          shift-right: [w334] -> w310
          shift-left: w313 -> [w335]
          tunnel: w312 -> [w333]
          shift-right: [w331] -> w309
          shift-left: w311 -> [w332]
          i -> [w345]
          n195 = call "tm_getnextframe_a.vi"("error in (no error)"=w353, "Buffer"=w354, "Handle in"=w355) -> ("error out"=w351:errorcluster, "Data"=w350:u16[][], "Handle out"=w352:u32)  [unwired: 6 in]
          n196 = call "ringbuffer.vi"("index in"=w332, "array size"=w333, "array in"=w335) -> ("index out"=w331:i32, "array out"=w334:dbl[])  [unwired: 7 in]
          n197 = Divide(x=w345, y=w344) -> (x/y=w343:dbl)
          n198 = case shown="True" w356 {
            tunnel: [w357 w360] -> w349
            tunnel: w350 -> [w357 w359]
            tunnel: w347 -> [_ w358]
            frame False {
            }
            frame True {
              n199 = Subtract(x=w359, y=w358) -> (x-y=w360:dbl[][])
            }
          }
          n200 = local write "Slide"(w343) -> ()
          n201 = call <vilib>:"Std Deviation and Variance.vi"("X"=w334) -> ("mean"=w336:dbl, "standard deviation"=w339:dbl)  [unwired: 1 in, 1 out]
          n202 = call "filtr_b.vi"("count?"=w346, "threshold"=w348, "input array"=w349) -> ("output array"=w341:dbl[][])  [unwired: 8 in]
          n203 = Divide(x=w339, y=w336) -> (x/y=w338:dbl)
          n204 = local write "live"(w341) -> ()
          n205 = Multiply(x=w338, y=100.0) -> (x*y=w340:dbl)
          n206 = local write "noise-o-meter"(w340) -> ()
          n207 = Add Array Elements(numeric array=w341) -> (sum=w342:dbl)
          n208 = local write "Waveform Chart"(w342) -> ()
        }
        n209 = call <vilib>:"Std Deviation and Variance.vi"("X"=w320) -> ("mean"=w317:dbl, "standard deviation"=w316:dbl)  [unwired: 1 in, 1 out]
        n210 = Format Into String(format string="%.6e;%.6e", w317, w316) -> (resulting string=w315:string)  [unwired: 2 in, 1 out]
        n211 = Enqueue Element(queue=w319, element=w315) -> ()  [unwired: 2 in, 3 out]
      }
      frame "dark" {
        n212 = Dequeue Element(queue=w367) -> ()  [unwired: 2 in, 4 out]
        n213 = local read "captured"() -> (w363:dbl[][])
      }
      frame "dark_load" {
        n214 = Dequeue Element(queue=w377) -> ()  [unwired: 2 in, 4 out]
        n215 = String To Path(string=w373) -> (path=w372:path)
        n216 = Read from Binary File(5:dbl[][] [] ("all rows"), 11:w372) -> (2:w370:dbl[][])  [unwired: 4 in, 3 out]
        n217 = call-poly <vilib>:"Read From Spreadsheet File.vi"("file path (dialog if empty)"=w372) -> ()  [unwired: 6 in, 5 out]
      }
      frame "release" {
        n218 = call "tm_stopcapture.vi"("error in (no error)"=w385, "Handle in"=w386) -> ("error out"=w383:errorcluster, "Handle out"=w384:u32)  [unwired: 8 in]
        n219 = Dequeue Element(queue=w389) -> ()  [unwired: 2 in, 4 out]
        n220 = call "tm_closecamera.vi"("error in (no error)"=w383, "Handle in"=w384) -> ("error out"=w382:errorcluster)  [unwired: 9 in]
        n221 = call "tm_deinitialize.vi"("error in (no error)"=w382) -> ("error out"=w381:errorcluster)  [unwired: 10 in]
      }
      frame "init" {
        n222 = Dequeue Element(queue=w392) -> ()  [unwired: 2 in, 4 out]
        n223 = call "tm_initialize.vi"() -> ("error out"=w398:errorcluster)  [unwired: 8 in, 3 out]
        n224 = call "tm_opencamera.vi"("error in (no error)"=w398, "Camera Index"=u32 0) -> ("error out"=w397:errorcluster, "Handle out"=w395:u32)  [unwired: 7 in, 1 out]
      }
      frame "set" {
        w424 = 1 items=["Snap", "Sequence"] ("Capture mode")
        w425 = u32 4215968 items=["BINNING"=4215968, "BITS PER CHANNEL"=2, "ACTIVE VIEW INDEX"=3, "CCD MODE"=4, "SENSOR MODE"=5, "READOUT MODE"=6, "EXPOSURE TIME"=7, "CONTRAST GAIN"=8, "CONTRAST OFFSET"=9, "LIGHT MODE"=10, "SENSITIVITY"=11, "WHITE BALANCE"=12, "PHOTON IMAGING MODE"=13, "HIGH DYNAMIC RANGE MODE"=14, "TRIGGER SOURCE"=15, "TRIGGER ACTIVE"=16, "TRIGGER MODE"=17, "TRIGGER POLARITY"=18, "TRIGGER GLOBAL EXPOSURE"=19, "FIRST TRIGGER BEHAVIOR"=20, "TRIGGER TIMES"=21, "OUTPUT TRIGGER POLARITY"=22, "OUTPUT TRIGGER DELAY"=23, "OUTPUT TRIGGER PERIOD"=24, "TEMPERATURE"=25, "TEMPERATURE TARGET"=26, "SENSOR COOLER FAN"=27, "MECHANICAL SHUTTER"=28, "BACK FOCUS POSITION"=29, "FRAMEBUNDLE MODE"=30, "FRAMEBUNDLE NUMBER"=31, "LINEBUNDLE HEIGHT"=32, "TRIGGER CONNECTOR"=33, "IMAGE PIXEL TYPE"=34, "OUTPUT TRIGGER KIND"=35, "READOUT DIRECTION"=36, "CHANNEL SYNC"=37] ("Parameter")
        w402 = u32 7 items=["BINNING"=4215968, "BITS PER CHANNEL"=2, "ACTIVE VIEW INDEX"=3, "CCD MODE"=4, "SENSOR MODE"=5, "READOUT MODE"=6, "EXPOSURE TIME"=7, "CONTRAST GAIN"=8, "CONTRAST OFFSET"=9, "LIGHT MODE"=10, "SENSITIVITY"=11, "WHITE BALANCE"=12, "PHOTON IMAGING MODE"=13, "HIGH DYNAMIC RANGE MODE"=14, "TRIGGER SOURCE"=15, "TRIGGER ACTIVE"=16, "TRIGGER MODE"=17, "TRIGGER POLARITY"=18, "TRIGGER GLOBAL EXPOSURE"=19, "FIRST TRIGGER BEHAVIOR"=20, "TRIGGER TIMES"=21, "OUTPUT TRIGGER POLARITY"=22, "OUTPUT TRIGGER DELAY"=23, "OUTPUT TRIGGER PERIOD"=24, "TEMPERATURE"=25, "TEMPERATURE TARGET"=26, "SENSOR COOLER FAN"=27, "MECHANICAL SHUTTER"=28, "BACK FOCUS POSITION"=29, "FRAMEBUNDLE MODE"=30, "FRAMEBUNDLE NUMBER"=31, "LINEBUNDLE HEIGHT"=32, "TRIGGER CONNECTOR"=33, "IMAGE PIXEL TYPE"=34, "OUTPUT TRIGGER KIND"=35, "READOUT DIRECTION"=36, "CHANNEL SYNC"=37] ("Parameter")
        n225 = Dequeue Element(queue=w418) -> ()  [unwired: 2 in, 4 out]
        n226 = call "tm_stopcapture.vi"("error in (no error)"=w432, "Handle in"=w430) -> ("error out"=w431:errorcluster, "Handle out"=w429:u32)  [unwired: 8 in]
        n227 = call "tm_unpreparecapture.vi"("error in (no error)"=w431, "Handle in"=w429) -> ("error out"=w428:errorcluster, "Handle out"=w427:u32)  [unwired: 8 in]
        n228 = call "tm_setparameter.vi"("error in (no error)"=w428, "Value in"="t_exp", "Parameter"=w402, "Handle in"=w427) -> ("error out"=w404:errorcluster, "Handle out"=w403:u32)  [unwired: 6 in]
        n229 = call "tm_getparameter.vi"("error in (no error)"=w404, "Parameter"=w402, "Handle in"=w403) -> ("error out"=w400:errorcluster, "Value out"=w399:dbl, "Handle out"=w401:u32)  [unwired: 6 in]
        n230 = local write "t_exp"(w399) -> ()
        n231 = call "tm_setparameter.vi"("error in (no error)"=w400, "Value in"="Value in", "Parameter"=w425, "Handle in"=w401) -> ("error out"=w408:errorcluster, "Handle out"=w409:u32)  [unwired: 6 in]
        n232 = call "tm_preparecapture.vi"("error in (no error)"=w408, "Frames"=1, "Capture mode"=w424, "Handle in"=w409) -> ("error out"=w421:errorcluster, "Buffer Info"=w420:T4, "Handle out"=w422:u32)  [unwired: 4 in, 1 out]
        n233 = call "tm_startcapture_b.vi"("error in (no error)"=w421, "Handle in"=w422) -> ("error out"=w406:errorcluster, "Handle out"=w407:u32)  [unwired: 8 in]
        n234 = Unbundle(w420) -> ("height"=w416:u32, "width"=w417:u32)  [unwired: 1 out]
        n235 = property on="live" class="IntGraph (strict)"("XScale.Minimum"=0.0 ("X Scale.Range:Minimum"), "XScale.Maximum"=w416, "YScale.Minimum"=0.0 ("Y Scale.Range:Minimum"), "YScale.Maximum"=w417) -> ()  [unwired: 2 in, 2 out]
        n236 = Initialize Array(u16 0 ("element"), w416, w417) -> (w419:u16[][])
      }
      frame "close" {
        n237 = Release Queue(queue=w440) -> ()  [unwired: 2 in, 3 out]
      }
    }
  }
  n238 = while {
    shift-right: [w443] -> _
    shift-left: _ -> [w451]
    shift-right: [w449] -> _
    shift-left: 200 -> [w450]
    shift-right: [w447] -> _
    shift-left: _ -> [w446]
    tunnel: w20 -> [w444]
    tunnel: w17 -> [w441]
    stop <- w452 stop-if-true
    # "ESP301"
    n239 = Preview Queue Element(queue=w441, timeout in ms (-1)=w450) -> (queue out=w448:refnum<queue>, element=w456:string)  [unwired: 1 in, 2 out]
    n240 = Match Pattern(string=w456, regular expression=":") -> (before substring=w454:string, after substring=w453:string)  [unwired: 1 in, 2 out]
    n241 = case shown="\"abs\"" w454 {
      tunnel: w453 -> [_ w481 w521 _ _ _]
      tunnel: [_ _ _ _ _ TRUE] -> w452
      tunnel: [w465 w476 w517 w524 w532 w537] -> w443
      tunnel: w451 -> [w468 w485 w519 w526 _ w537]
      tunnel: w448 -> [_ w472 w513 w523 w533 w535]
      tunnel: [w466 w469 w518 refnum<visa-resource-name> refnum ("VISA resource name out") w531 w536] -> w447
      tunnel: w446 -> [w467 w484 w520 w527 _ w536]
      tunnel: "esp_axis" -> [w464 w470 w516 _ _ _]
      tunnel: w444 -> [_ w474 _ _ _ _]
      tunnel: [200 0 0 0 0 0] -> w442
      frame "idle", Default {
        n242 = call "Read Actual Position.vi"("error in (no error)"=w468, "Axis (1)"=w464, "VISA resource name"=w467) -> ("error out"=w465:errorcluster, "Position (units)"=w459:dbl, "VISA resource name out"=w466:refnum<visa-resource-name>)  [unwired: 2 in]
        n243 = local read "t0 @"() -> (w462:dbl)
        n244 = call "mm2time.vi"("fs?"=TRUE, "Offset (mm)"=w462, "distance (mm)"=w459) -> ("time in fs/ps seconds"=w460:dbl)
        n245 = local write "delay_pos"(w459) -> ()
        n246 = local write "esp_pos_fs"(w460) -> ()
      }
      frame "abs" {
        n247 = Dequeue Element(queue=w472) -> ()  [unwired: 2 in, 4 out]
        n248 = Match Pattern(string=w481, regular expression=":") -> (before substring=w480:string, after substring=w479:string)  [unwired: 1 in, 2 out]
        n249 = Equal?(x=w479, y="confirm") -> (x = y?=w475:bool)
        n250 = Fract/Exp String To Number(string=w480) -> (number=w483:dbl)  [unwired: 3 in, 1 out]
        n251 = call "Move Absolute.vi"("error in (no error)"=w485, "Position (0 units)"=w483, "Axis (1)"=w470, "VISA resource name"=w484) -> ("error out"=w477:errorcluster, "VISA resource name out"=w471:refnum<visa-resource-name>)  [unwired: 2 in]
        n252 = case shown="True" w475 {
          tunnel: w477 -> [w487 w492]
          tunnel: [w487 w495] -> w476
          tunnel: w474 -> [_ w494]
          tunnel: w471 -> [w486 w490]
          tunnel: w470 -> [_ w489]
          tunnel: [w486 w488] -> w469
          frame False {
          }
          frame True {
            n253 = while {
              tunnel: w490 -> [w500]
              tunnel: w489 -> [w496]
              shift-right: [w504] -> w491
              shift-left: w492 -> [w499]
              tunnel: [w503] -> w488
              stop <- w506 continue-if-true
              n254 = call "Read Actual Position.vi"("error in (no error)"=w499, "Axis (1)"=w496, "VISA resource name"=w500) -> ("error out"=w497:errorcluster, "Position (units)"=w501:dbl, "VISA resource name out"=w498:refnum<visa-resource-name>)  [unwired: 2 in]
              n255 = local write "delay_pos"(w501) -> ()
              n256 = Decrement(x=w496) -> (x-1=w502:i32)
              n257 = call "Get Controller Status.vi"("error in (no error)"=w497, "VISA resource name"=w498) -> ("error out"=w504:errorcluster, "Controller Status"=w512:T5, "VISA resource name out"=w503:refnum<visa-resource-name>)  [unwired: 2 in, 1 out]
              n258 = Unbundle(w512) -> ("Axis1 moving"=w511:bool, "Axis2 moving"=w510:bool, "Axis3 moving"=w509:bool, "Axis4 moving"=w508:bool)  [unwired: 12 out]
              n259 = Build Array(w511, w510, w509, w508) -> (w507:bool[])
              n260 = Index Array(array=w507, index=w502) -> (element=w505:bool)
              n261 = Or(x=w505, y=w504) -> (x .or. y?=w506:bool)
            }
            n262 = Send Notification(notification=TRUE, notifier=w494, error in (no error)=w491) -> (error out=w495:errorcluster)  [unwired: 1 out]
          }
        }
      }
      frame "rel" {
        n263 = Dequeue Element(queue=w513) -> ()  [unwired: 2 in, 4 out]
        n264 = Fract/Exp String To Number(string=w521) -> (number=w515:dbl)  [unwired: 3 in, 1 out]
        n265 = call "Move Relative.vi"("error in (no error)"=w519, "Position (0 units)"=w515, "Axis (1)"=w516, "VISA resource name"=w520) -> ("error out"=w517:errorcluster, "VISA resource name out"=w518:refnum<visa-resource-name>)  [unwired: 2 in]
      }
      frame "release" {
        n266 = Dequeue Element(queue=w523) -> ()  [unwired: 2 in, 4 out]
        n267 = call "Close.vi"("error in (no error)"=w526, "VISA resource name"=w527) -> ("error out"=w524:errorcluster)  [unwired: 9 in]
      }
      frame "init" {
        n268 = Dequeue Element(queue=w533) -> ()  [unwired: 2 in, 4 out]
        n269 = call "Initialize.vi"("VISA resource name"="esp_visa", "Serial Link (RS232)"="Serial Link (RS232)") -> ("VISA resource name out"=w531:refnum<visa-resource-name>, "error out"=w532:errorcluster)  [unwired: 7 in]
      }
      frame "close" {
        n270 = Release Queue(queue=w535) -> ()  [unwired: 2 in, 3 out]
      }
    }
    "esp301" <- w443
    n271 = case shown="No Error" w443 {
      tunnel: [w457 -1] -> w449
      tunnel: w442 -> [w457 _]
      frame No Error {
      }
      frame Error {
      }
    }
  }
  n272 = while {
    tunnel: w25 -> [w547]
    shift-right: [w545] -> _
    shift-left: _ -> [w544]
    shift-right: [w542] -> _
    shift-left: -1 -> [w543]
    shift-right: [w541] -> _
    shift-left: _ -> [w540]
    tunnel: w23 -> [w539]
    stop <- w546 stop-if-true
    # "ISEG"
    n273 = Preview Queue Element(queue=w547, timeout in ms (-1)=w543) -> (element=w551:string)  [unwired: 1 in, 3 out]
    n274 = Match Pattern(string=w551, regular expression=":") -> (before substring=w549:string, after substring=w548:string)  [unwired: 1 in, 2 out]
    n275 = case shown="\"set\"" w549 {
      tunnel: w548 -> [_ w565 _ _ _]
      tunnel: w547 -> [_ w577 w619 w623 w627]
      tunnel: [_ _ _ _ TRUE] -> w546
      tunnel: [w554 w571 w617 w622 w624] -> w545
      tunnel: w544 -> [w556 w575 _ _ w624]
      tunnel: [0 _ _ _ _] -> w542
      tunnel: [w555 w572 T6 {"VISA Resource Name"="", "FP Notation"=FALSE, "Maximum Voltage"=0, "Maximum Current"=0} ("VISA Session Out") w620 w625] -> w541
      tunnel: w540 -> [w557 w576 w618 _ w625]
      tunnel: w539 -> [_ w560 _ _ _]
      frame "idle", Default {
        n276 = local read "Channel (A)"() -> (w558:enum16{"A", "B"})
        n277 = call "iseg NHQ xxx GetActualVoltage.vi"("error in (no error)"=w556, "Channel (A)"=w558, "VISA Session"=w557) -> ("error out"=w554:errorcluster, "Voltage"=w553:dbl, "VISA Session Out"=w555:T6)  [unwired: 5 in, 1 out]
        n278 = node(w553) -> (w552:dbl[unit])
        n279 = local write "Actual Voltage"(w552) -> ()
      }
      frame "set" {
        n280 = local read "Channel (A)"() -> (w568:enum16{"A", "B"})
        n281 = Dequeue Element(queue=w577) -> ()  [unwired: 2 in, 4 out]
        n282 = Match Pattern(string=w565, regular expression=":") -> (before substring=w564:string, after substring=w563:string)  [unwired: 1 in, 2 out]
        n283 = Fract/Exp String To Number(string=w564) -> (number=w567:dbl)  [unwired: 3 in, 1 out]
        n284 = call "iseg NHQ xxx SetNominalVoltage.vi"("error in (no error)"=w575, "Voltage (0 V)"=w567, "Channel (A)"=w568, "VISA Session"=w576) -> ("error out"=w578:errorcluster, "VISA Session Out"=w579:T6)  [unwired: 6 in]
        n285 = Equal?(x=w563, y="wait") -> (x = y?=w561:bool)
        n286 = call "iseg NHQ xxx StartVoltageChange.vi"("error in (no error)"=w578, "Channel (A)"=w568, "VISA Session"=w579) -> ("error out"=w573:errorcluster, "VISA Session Out"=w574:T6)  [unwired: 6 in, 1 out]
        n287 = case shown="True" w561 {
          tunnel: [w581 w591] -> w572
          tunnel: [w580 w583] -> w571
          tunnel: w574 -> [w581 w590]
          tunnel: w573 -> [w580 w589]
          tunnel: w567 -> [_ w588]
          tunnel: "volt_threshold" -> [_ w587]
          tunnel: "volt_timeout" -> [_ w586]
          tunnel: w568 -> [_ w585]
          tunnel: w560 -> [_ w584]
          frame False {
          }
          frame True {
            n288 = Tick Count (ms)() -> (millisecond timer value=w592:u32)
            n289 = while {
              shift-right: [w613] -> w591
              shift-left: w590 -> [w615]
              shift-right: [w600] -> w583
              shift-left: w589 -> [w614]
              tunnel: w585 -> [w612]
              tunnel: w587 -> [w609]
              tunnel: w592 -> [w607]
              tunnel: w586 -> [w605]
              tunnel: w588 -> [w604]
              tunnel: [w595] -> w582
              stop <- w601 stop-if-true
              n290 = Tick Count (ms)() -> (millisecond timer value=w608:u32)
              n291 = call "iseg NHQ xxx GetActualVoltage.vi"("error in (no error)"=w614, "Channel (A)"=w612, "VISA Session"=w615) -> ("error out"=w600:errorcluster, "Voltage"=w593:dbl, "VISA Session Out"=w613:T6)  [unwired: 5 in, 1 out]
              n292 = Absolute Value(x=w593) -> (abs(x)=w603:dbl)
              n293 = node(w593) -> (w594:dbl[unit])
              n294 = Subtract(x=w608, y=w607) -> (x-y=w606:u32)
              n295 = Subtract(x=w603, y=w604) -> (x-y=w611:dbl)
              n296 = local write "Actual Voltage"(w594) -> ()
              n297 = Absolute Value(x=w611) -> (abs(x)=w610:dbl)
              n298 = Greater?(x=w606, y=w605) -> (0:w599:bool)
              n299 = Less?(x=w610, y=w609) -> (x < y?=w602:bool)
              n300 = Or(x=w600, y=w599) -> (x .or. y?=w598:bool)
              n301 = Compound Arithmetic op=OR(w600, w602, w599) -> (w601:bool)
              n302 = Select(t="fail" ("element"), s=w598, f="done" ("element")) -> (s? t:f=w595:string)
            }
            n303 = Enqueue Element(queue=w584, element=w582) -> ()  [unwired: 2 in, 3 out]
          }
        }
      }
      frame "release" {
        n304 = Dequeue Element(queue=w619) -> ()  [unwired: 2 in, 4 out]
        n305 = call "iseg NHQ xxx Close.vi"("VISA session"=w618) -> ("error out"=w617:errorcluster)  [unwired: 14 in]
      }
      frame "init" {
        n306 = Dequeue Element(queue=w623) -> ()  [unwired: 2 in, 4 out]
        n307 = call "iseg NHQ xxx Initialize.vi"("VISA resource name"="VISA ISEG") -> ("VISA Session Out"=w620:T6, "error out"=w622:errorcluster)  [unwired: 13 in]
      }
      frame "close" {
        n308 = Release Queue(queue=w627) -> ()  [unwired: 2 in, 3 out]
      }
    }
    "error out" <- w545
  }
  n309 = while {
    tunnel: w23 -> [w636]
    tunnel: w31 -> [w635]
    tunnel: w30 -> [w633]
    tunnel: w25 -> [w632]
    tunnel: w6 -> [w631]
    tunnel: w20 -> [w630]
    tunnel: w17 -> [w629]
    tunnel: w1 -> [w628]
    stop <- w634 stop-if-true
    # "coherent"
    n310 = Preview Queue Element(queue=w636) -> (element=w640:string)  [unwired: 2 in, 3 out]
    n311 = Match Pattern(string=w640, regular expression=":") -> (before substring=w638:string, after substring=w637:string)  [unwired: 1 in, 2 out]
    n312 = case shown="\"delay\"" w638 {
      tunnel: w637 -> [_ _ _ _ _]
      tunnel: w636 -> [w642 w648 w673 w757 _]
      tunnel: w635 -> [w643 w644 w665 w755 _]
      tunnel: [TRUE _ _ _ _] -> w634
      tunnel: w633 -> [_ w647 w666 w754 _]
      tunnel: w632 -> [_ _ w667 _ _]
      tunnel: w631 -> [_ _ w668 _ _]
      tunnel: w630 -> [_ _ _ w771 _]
      tunnel: w629 -> [_ _ _ w752 _]
      tunnel: w628 -> [_ _ _ _ _]
      frame "close" {
        n313 = Release Queue(queue=w642) -> ()  [unwired: 2 in, 3 out]
        n314 = Release Queue(queue=w643) -> ()  [unwired: 2 in, 3 out]
      }
      frame "single" {
        n315 = Dequeue Element(queue=w648) -> (error out=w645:errorcluster)  [unwired: 2 in, 3 out]
        n316 = Flush Queue(queue=w644, error in (no error)=w645) -> (error out=w646:errorcluster)  [unwired: 2 out]
        n317 = while {
          tunnel: w647 -> [w652]
          tunnel: w646 -> [w651]
          tunnel: w644 -> [w650]
          stop <- w649 continue-if-true
          n318 = flat-sequence {
            tunnel: w652 -> [w657]
            tunnel: w651 -> [w654]
            tunnel: w650 -> [w653]
            tunnel: ["continous acq."] -> w649
            frame #0 {
              n319 = Enqueue Element(queue=w657, element="snap", error in (no error)=w654) -> (error out=w655:errorcluster)  [unwired: 1 in, 2 out]
              n320 = Dequeue Element(queue=w653, error in (no error)=w655) -> ()  [unwired: 1 in, 4 out]
            }
            frame #1 {
            }
          }
        }
      }
      frame "volt" {
        n321 = Flush Queue(queue=w673) -> (queue out=w669:refnum<queue>)  [unwired: 1 in, 2 out]
        n322 = local read "Path"() -> (w672:path)
        n323 = Build Path(base path=w672, name or relative path="head") -> (appended path=w660:path)
        n324 = Build Path(base path=w660, name or relative path="raw") -> (appended path=w662:path)
        n325 = Build Path(base path=w660, name or relative path="LUT.txt") -> (appended path=w663:path)
        n326 = Create Folder(path (use dialog)=w662) -> (created path=w661:path)  [unwired: 2 in, 2 out]
        n327 = while {
          tunnel: w669 -> [w674]
          tunnel: w668 -> [w697]
          tunnel: w667 -> [w691]
          tunnel: w666 -> [w690]
          tunnel: w665 -> [w689]
          tunnel: w663 -> [w684]
          tunnel: w661 -> [w683]
          shift-right: [w676] -> _
          shift-left: _ -> [w681]
          tunnel: [w674] -> w659
          i -> [w688]
          stop <- w675 stop-if-true
          n328 = call-poly <vilib>:"Ramp Pattern.vi"("start"="volt_start", "end"="volt_end", "samples"="volt_samples") -> ("Ramp Pattern"=w687:dbl[])  [unwired: 7 in, 1 out]
          n329 = Array Size(array=w687) -> (size(s)=w686:i32)
          n330 = Number To Fractional String(number=w687) -> (F-format string=w693:string[])  [unwired: 3 in]
          n331 = Multiply(x=w686, y=w688) -> (x*y=w685:i32)
          n332 = for {
            N -> [w700]
            tunnel: w697 -> [w727]
            tunnel: w674 -> [w734]
            tunnel: w693 -> [w717] mode=indexing
            tunnel: "set:" ("element") -> [w731]
            tunnel: w691 -> [w730]
            tunnel: w674 -> [w728]
            tunnel: w690 -> [w725]
            tunnel: w689 -> [w722]
            shift-right: [w702] -> w682
            shift-left: w681 -> [w720]
            tunnel: w685 -> [w719]
            tunnel: w684 -> [w716]
            tunnel: w683 -> [w715]
            tunnel: ":wait" ("element") -> [w701]
            i -> [w699]
            n333 = Concatenate Strings(w731, w717, w701) -> (w732:string)
            n334 = Add(x=w719, y=w699) -> (x+y=w718:i32)
            n335 = Divide(x=w699, y=w700) -> (x/y=→"Slide 2":dbl)
            n336 = Number To Decimal String(number=w718) -> (decimal integer string=w714:string)  [unwired: 1 in]
            n337 = Enqueue Element(queue=w730, element=w732, error in (no error)=w720) -> (error out=w729:errorcluster)  [unwired: 1 in, 2 out]
            n338 = Dequeue Element(queue=w728, error in (no error)=w729) -> (element=w711:string, error out=w709:errorcluster)  [unwired: 1 in, 2 out]
            n339 = Equal?(x="stop" ("y"), y=w711) -> (x = y?=w708:bool)
            n340 = call "inject_error.vi"("error in"=w709, "s"=w708) -> ("error out"=w710:errorcluster)  [unwired: 9 in]
            n341 = Enqueue Element(queue=w727, element="start", error in (no error)=w710) -> (error out=w724:errorcluster)  [unwired: 1 in, 2 out]
            n342 = Enqueue Element(queue=w725, element="snap", error in (no error)=w724) -> (error out=w723:errorcluster)  [unwired: 1 in, 2 out]
            n343 = Dequeue Element(queue=w722, error in (no error)=w723) -> (element=w713:dbl[][], error out=w721:errorcluster)  [unwired: 1 in, 2 out]
            n344 = Enqueue Element(queue=w727, element="ok", error in (no error)=w721) -> (error out=w733:errorcluster)  [unwired: 1 in, 2 out]
            n345 = Dequeue Element(queue=w734, error in (no error)=w733) -> (element=w705:string, error out=w704:errorcluster)  [unwired: 1 in, 2 out]
            n346 = Equal?(x="stop" ("y"), y=w705) -> (x = y?=w707:bool)
            n347 = call "inject_error.vi"("error in"=w704, "s"=w707) -> ("error out"=w703:errorcluster)  [unwired: 9 in]
            n348 = case shown="No Error" w703 {
              selector: w703 -> [w740 w750]
              tunnel: w717 -> [w739 _]
              tunnel: w716 -> [w746 _]
              tunnel: w715 -> [w745 _]
              tunnel: w714 -> [w744 _]
              tunnel: w713 -> [w742 _]
              tunnel: w705 -> [w741 _]
              tunnel: [w740 w750] -> w702
              frame No Error {
                n349 = Build Path(base path=w745, name or relative path=w744) -> (appended path=w743:path)
                n350 = Match Pattern(string=w741, regular expression=";") -> (before substring=w747:string, after substring=w738:string)  [unwired: 1 in, 2 out]
                n351 = Write to Binary File(file (use dialog)=w743, data=w742) -> ()  [unwired: 4 in, 3 out]
                n352 = Build Array(w744, w747, w738, w739) -> (w737:string[])
                n353 = call-poly <vilib>:"Write Delimited Spreadsheet.vi"("file path (dialog if empty)"=w746, "1D data"=w737, "append to file? (new file:F)"=TRUE) -> ()  [unwired: 11 in, 2 out]
              }
              frame Error {
              }
            }
          }
          n354 = Dequeue Element(queue=w674, error in (no error)=w682) -> (element=w679:string, error out=w676:errorcluster)  [unwired: 1 in, 2 out]
          n355 = Equal?(x="stop" ("y"), y=w679) -> (x = y?=w677:bool)
          n356 = Or(x=w677, y=w676) -> (x .or. y?=w675:bool)
        }
        n357 = Flush Queue(queue=w659) -> ()  [unwired: 1 in, 3 out]
      }
      frame "delay" {
        n358 = local read "Path"() -> (w770:path)
        n359 = Dequeue Element(queue=w757) -> ()  [unwired: 2 in, 4 out]
        n360 = Build Path(base path=w770, name or relative path="delayscan_header") -> (appended path=w759:path)
        n361 = call <vilib>:"Check if File or Folder Exists.vi"("path"=w759) -> ("file or folder exists?"=w761:bool, "dup path"=w760:path)  [unwired: 8 in, 1 out]
        n362 = case shown="False" w761 {
          tunnel: [w886 w887] -> w758
          tunnel: w760 -> [w885 w887]
          frame False {
            n363 = Create Folder(path (use dialog)=w885) -> (created path=w886:path)  [unwired: 2 in, 2 out]
          }
          frame True {
          }
        }
        n364 = call "create scan vectr.vi"("Table Control"="waypoints") -> ("Array"=w762:dbl[])
        n365 = Flush Queue(queue=w755) -> (queue out=w756:refnum<queue>)  [unwired: 1 in, 2 out]
        n366 = Array Size(array=w762) -> (size(s)=w765:i32)
        n367 = Build Path(base path=w758, name or relative path="times.txt") -> (appended path=w767:path)
        n368 = Flush Queue(queue=w752) -> (queue out=w751:refnum<queue>)  [unwired: 1 in, 2 out]
        n369 = Flush Queue(queue=w754) -> (queue out=w753:refnum<queue>)  [unwired: 1 in, 2 out]
        n370 = Initialize Array(0.0 ("element"), w765) -> (w763:dbl[])
        n371 = call-poly <vilib>:"Write Delimited Spreadsheet.vi"("file path (dialog if empty)"=w767, "1D data"=w762, "transpose? (no:F)"=TRUE) -> ()  [unwired: 11 in, 2 out]
        n372 = while {
          tunnel: w762 -> [w783]
          tunnel: w751 -> [w787]
          tunnel: w771 -> [w786]
          tunnel: w756 -> [w785]
          tunnel: w753 -> [w784]
          tunnel: w758 -> [w782]
          shift-right: [w780] -> _
          shift-left: w763 -> [w781]
          tunnel: w758 -> [w779]
          i -> [w776]
          stop <- w773 stop-if-true
          n373 = for {
            tunnel: w783 -> [w788] mode=indexing
            tunnel: w787 -> [w856]
            tunnel: w786 -> [w854]
            tunnel: w785 -> [w852]
            tunnel: w784 -> [w850]
            tunnel: w783 -> [w820]
            tunnel: w782 -> [w848]
            tunnel: w776 -> [w797]
            shift-right: [w818] -> w780
            shift-left: w781 -> [w821]
            tunnel: w779 -> [w816]
            tunnel: ["delayscan_stop"] -> w775
            i -> [w801]
            stop <- "delayscan_stop" stop-if-true
            n374 = local read "t0 @"() -> (w861:dbl)
            n375 = Get Date/Time In Seconds() -> (seconds since 1Jan1904=w793:timestamp)
            n376 = Divide(x=w797, y=10000) -> (x/y=w846:dbl)
            n377 = Format Date/Time String(time format string (%c)="DelayScan_%Y%m%d_%H%M%S_", seconds (now)=w793) -> (date/time string=w789:string)  [unwired: 1 in]
            n378 = Divide(x=w801, y=10000) -> (x/y=w800:dbl)
            n379 = Number To Fractional String(number=w846) -> (F-format string=w845:string)  [unwired: 3 in]
            n380 = call "time2mm.vi"("fs[1]/ps[0]"=TRUE, "Offset (mm)"=w861, "time"=w788) -> ("position (mm)"=w796:dbl)
            n381 = Number To Fractional String(number=w800) -> (F-format string=w841:string)  [unwired: 3 in]
            n382 = Number To Fractional String(number=w796) -> (F-format string=w859:string)  [unwired: 3 in]
            n383 = String Subset(string=w845, offset (0)=2, length (rest)=4 ("length (rest)")) -> (substring=w843:string)
            n384 = String Subset(string=w841, offset (0)=2, length (rest)=4 ("length (rest)")) -> (substring=w791:string)
            n385 = Concatenate Strings("abs:" ("string"), w859, ":confirm" ("string")) -> (w857:string)
            n386 = Build Path(base path=w848, name or relative path=w843) -> (appended path=w804:path)
            n387 = call <vilib>:"Check if File or Folder Exists.vi"("path"=w804) -> ("file or folder exists?"=w805:bool, "dup path"=w806:path)  [unwired: 8 in, 1 out]
            n388 = Concatenate Strings(w789, w791) -> (w792:string)
            n389 = case shown="False" w805 {
              tunnel: [w883 w884] -> w803
              tunnel: w806 -> [w882 w884]
              frame False {
                n390 = Create Folder(path (use dialog)=w882) -> (created path=w883:path)  [unwired: 2 in, 2 out]
              }
              frame True {
              }
            }
            n391 = Enqueue Element(queue=w856, element=w857) -> (error out=w855:errorcluster)  [unwired: 2 in, 2 out]
            n392 = Concatenate Strings(w792, ".bin" ("string")) -> (w811:string)
            n393 = Concatenate Strings(w792, ".png" ("string")) -> (w809:string)
            n394 = Wait on Notification(notifier=w854, error in (no error)=w855) -> (error out=w853:errorcluster)  [unwired: 2 in, 3 out]
            n395 = Build Path(base path=w803, name or relative path=w811) -> (appended path=w817:path)
            n396 = Build Path(base path=w816, name or relative path="positions.txt") -> (appended path=w814:path)
            n397 = property on="live" class="IntGraph (strict)"() -> ("CrsrLis"=w840:T7)  [unwired: 2 in, 2 out]
            n398 = Build Path(base path=w803, name or relative path=w809) -> (appended path=w808:path)
            n399 = Enqueue Element(queue=w850, element="snap", error in (no error)=w853) -> (error out=w851:errorcluster)  [unwired: 1 in, 2 out]
            n400 = Index Array(array=w840) -> (element #1=w839:T8, element #2=w838:T8)  [unwired: 2 in]
            n401 = Unbundle By Name(w839) -> ("Position.X"=w837:dbl, "Position.Y"=w835:dbl)
            n402 = Unbundle By Name(w838) -> ("Position.X"=w836:dbl, "Position.Y"=w834:dbl)
            n403 = Dequeue Element(queue=w852, error in (no error)=w851) -> (element=w807:dbl[][])  [unwired: 1 in, 3 out]
            n404 = Build Array(w837, w836) -> (w833:dbl[])
            n405 = Build Array(w835, w834) -> (w832:dbl[])
            n406 = Array Max & Min(array=w833) -> (max value=w831:dbl, min value=w829:dbl)  [unwired: 2 out]
            n407 = Array Max & Min(array=w832) -> (max value=w830:dbl, min value=w827:dbl)  [unwired: 2 out]
            n408 = Write to Binary File(file (use dialog)=w817, data=w807) -> ()  [unwired: 4 in, 3 out]
            n409 = Subtract(x=w829, y=w831) -> (x-y=w828:dbl)
            n410 = Subtract(x=w827, y=w830) -> (x-y=w826:dbl)
            n411 = Array Subset(array=w807, index (row)=w829, length (row)=w828, index (col)=w827, length (col)=w826) -> (w825:dbl[][])
            n412 = Array Size(array=w807) -> (size(s)=w823:i32[])
            n413 = Add Array Elements(numeric array=w825) -> (sum=w824:dbl)
            n414 = Multiply Array Elements(1:w823) -> (0:w822:i32)
            n415 = Divide(x=w824, y=w822) -> ()  [unwired: 1 out]
            n416 = disable-structure shown="Disabled" {
              disable-tunnel: w808 -> [w864 _]
              disable-tunnel: w807 -> [w863 _]
              frame Disabled {
                w878 = T2 7 items=["Grayscale (U8)", "Grayscale (I16)", "Grayscale (SGL)", "Complex (CSG)", "RGB (U32)", "HSL (U32)", "RGB (U64)", "Grayscale (U16)"] ("Image Type")
                n417 = for {
                  tunnel: w863 -> [w881] mode=indexing
                  tunnel: [w880] -> w873 mode=indexing
                  n418 = Reverse 1D Array(array=w881) -> (reversed array=w880:dbl[])
                }
                n419 = Transpose 2D Array(2D array=w873) -> (transposed array=w867:dbl[][])
                n420 = Array Max & Min(array=w867) -> (min value=w866:dbl)  [unwired: 3 out]
                n421 = Subtract(x=w867, y=w866) -> (x-y=w865:dbl[][])
                n422 = call "IMAQ Create"("Image Name"="untitled", "Image Type"=w878) -> ("New Image"=w879:T3)  [unwired: 3 in, 1 out]
                n423 = Array Max & Min(array=w865) -> (max value=w872:dbl)  [unwired: 3 out]
                n424 = Divide(x=w865, y=w872) -> (x/y=w871:dbl[][])
                n425 = Multiply(x=w871, y=255) -> (x*y=w869:dbl[][])
                n426 = To Unsigned Word Integer(number=w869) -> (unsigned 16bit integer=w868:u16[][])
                n427 = call "IMAQ ArrayToImage"("Image Pixels (U16)"=w868, "Image"=w879) -> ("Image Out"=w877:T3)  [unwired: 8 in, 1 out]
                n428 = call-poly "IMAQ Write File 2"("Image Quality"=u32 1000, "File Path"=w864, "Image"=w877) -> ("Image Out (duplicate)"=w875:T3)  [unwired: 7 in, 1 out]
                n429 = call "IMAQ Dispose"("Image"=w875) -> ()  [unwired: 5 in, 1 out]
              }
              frame Enabled {
              }
            }
            n430 = Replace Array Subset(array=w821, new element=w796, index=w801) -> (w818:dbl[])
            n431 = Bundle("Array"=w820, w818) -> (→"XY Graph":cluster{"Array":dbl[], dbl[]})  [unwired: 1 in]
            n432 = call-poly <vilib>:"Write Delimited Spreadsheet.vi"("file path (dialog if empty)"=w814, "format (%.3f)"="%.6f", "1D data"=w818, "transpose? (no:F)"=TRUE) -> ()  [unwired: 10 in, 2 out]
          }
          n433 = Increment(x=w776) -> (x+1=w777:i32)
          n434 = Greater Or Equal?(x=w777, y="iterations") -> (x >= y?=w774:bool)
          n435 = Or(x=w775, y=w774) -> (x .or. y?=w773:bool)
        }
      }
      frame "idle", Default {
      }
    }
  }
